vi "RH_Auto_with_Lockin_clear.vi"() -> ()   [LabVIEW 2019]
uses:
  <vilib>/Instr/_visa.llb/VISA Configure Serial Port (Instr).vi
  <vilib>/ptbypt/NI_PtbyPt.lvlib
panel:
  in  "0:OFF\n1:2.5mW\n2:25mW\n3:250mW\n4:2.5W\n5:25W":dbl=3.0
  in  "1:VTI 2:Sample":dbl=2.0
  in  "Termination Character":u8=10 format="%.0x"
  in  "Set VTI Heater Range":bool
  in  "Apply voltage":bool
  out "read buffer":string
  in  "Target [V]":string
  in  "start [V]":string
  in  "Keithley2400":refnum<visa-resource-name>="GPIB1::15::INSTR"
  out "Resistance [Ohm]":dbl=97.3586 format="%#_6f"
  out "Lockin y (V)":dbl=136.05
  out "Lockin x (V)":dbl=0.000139774
  in  "On:Delta\nOff:Lock-in":bool=TRUE
  in  "I for Lockin [A]":dbl=5e-06 format="%#_6e"
  out "Lockin Y (V)":dbl=-136.536
  out "Lockin X (V)":dbl=0.000486793
  in  "Lockin SR830":refnum<visa-resource-name>="GPIB1::8::INSTR"
  in  "T-ramp off":bool
  in  "Main sorb T control":bool
  in  "Wait [min]":i32
  in  "LakeShore335 (for He3)":refnum<visa-resource-name>="COM4"
  in  "Temp control off":bool
  out "temp [K]":dbl=1.4
  out "Waiting T-stability":bool caption="stabilizing"
  in  "Set Initial Field":bool
  in  "Field [T]":dbl
  in  "Period [s]":dbl=0.5 caption="Delay Time (s)"
  in  "Measure R-T":bool
  in  "Save R-T":bool
  out "R-T":cluster{"X":dbl[], "Y":dbl[]}[](graph) caption="XY Graph"
  out "Rate [K/min]":dbl=-0.11815951044220217 format="%#_6f"
  in  "Reset":bool
  in  "Stop":bool
  in  "Pause off":bool
  in  "Compliance [V]":dbl=0.5 format="%#_6f"
  out "R-H":cluster{"X":dbl[], "Y":dbl[]}[](graph) caption="XY Graph"
  in  "Reset":bool
  in  "Folder":path=path "C:/User Data/Graham" caption="Filename"
  out "Filename Out":path=path "C:/User Data/Bart/CG014_1012_3.00K"
  in  "File name":string="CG017a_3uA"
  out "VTI [K]":dbl=3.087
  out "VTI [K]":dbl=1.6151
  out "Sample Temp [K]":dbl=1.4
  out "Magnetic Field [T]":dbl=2.97271
  out "Delta reading [Ohm]":dbl
  out "Delta Reading [Ohm]":dbl=0.00314207515
  out "Sample Temp [K]":dbl=2.2127
  in  "Abort Delta":bool
  in  "Arm Delta":bool
  in  "DELAY [sec]":dbl=0.002 format="%#_6e"
  in  "I-HIGH [A]":dbl=0.0001 format="%#_6e"
  in  "Measure R-H":bool
  in  "Rate [K/min]":dbl=10.0
  in  "Set Temp [K]":dbl=1.0
  in  "Set Temperature":bool
  out "Magnetic Field [T]":dbl
  in  "Rate [T/min]":dbl=0.5
  in  "Set Field [T]":dbl
  in  "Set Field":bool
  in  "Keithley":refnum<visa-resource-name>="GPIB1::20::INSTR"
  in  "Skip":bool
  in  "Wait T-stable [min]":i32=30
  in  "period (s)":dbl=0.5 min=0.0 max=1111.0 step=0.1
  in  "stop 2":bool caption="Pause"
  in  "Wait field stable [sec]":dbl=20.0
  in  "Magnet Power supply":refnum<visa-resource-name>="COM6"
  in  "Set Field [T]   Rate [T/min]":dbl[][](array[numeric])=[[0.0, 0.2], [-6.0, 0.2], [0.0, 0.2], [6.0, 0.2]]
  in  "Set Temp [K]  Rate [K/min]":dbl[][](array[numeric])=[[10.0, 5.0], [0.0, 5.0], [0.0, 5.0], [0.0, 5.0], [0.0, 5.0]]
  in  "LakeShore340":refnum<visa-resource-name>="COM7"
  out "error out 3":errorcluster={"status"=FALSE, "code"=1073676294, "source"="VISA Read in RH_Auto_with_Lockin_clear.vi"}
  out "error out 2":errorcluster={"status"=FALSE, "code"=1073676294, "source"="VISA Read in RH_Auto_with_Lockin_clear.vi"}
  out "error out":errorcluster={"status"=FALSE, "code"=1073676294, "source"="VISA Read in RH_Auto_with_Lockin_clear.vi"}
  # "Manual control"
  # "R-H Auto Measurement"
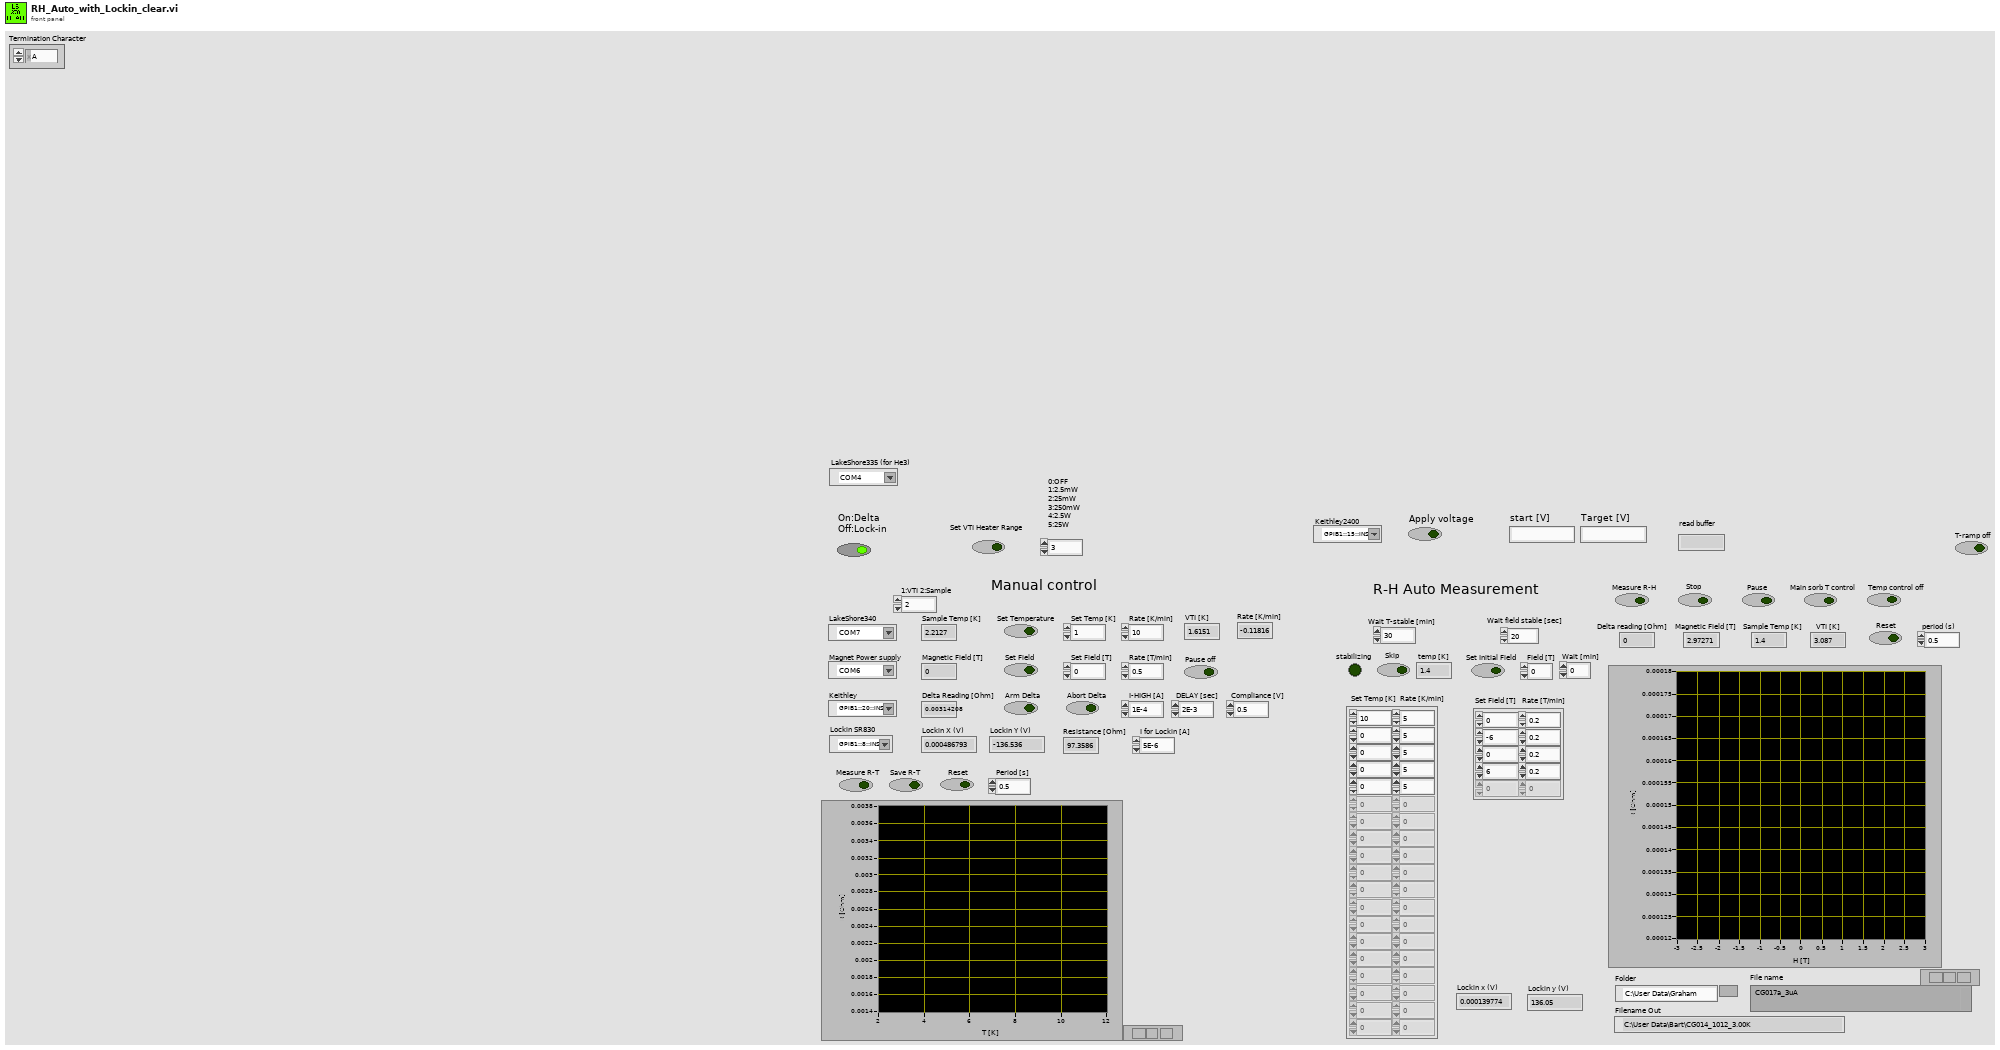
[diagram p1: front panel]
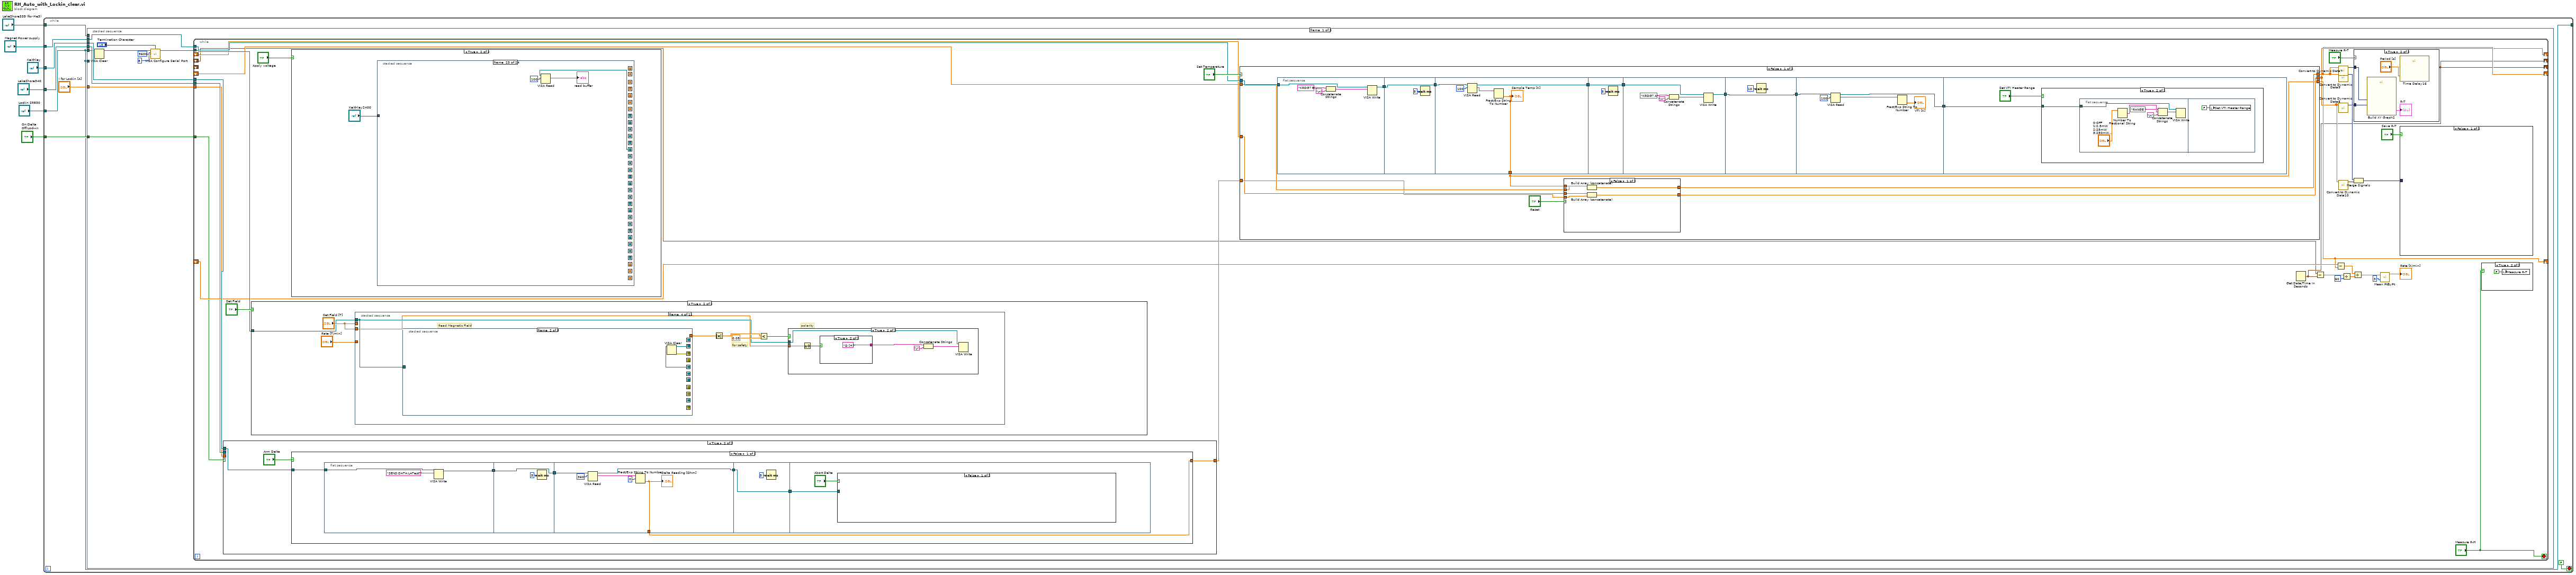
[diagram p0: block diagram]
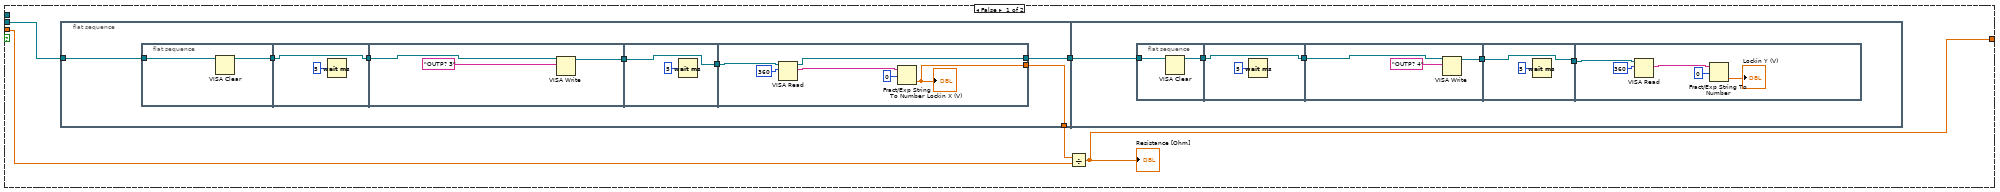
[diagram p2: hidden frame]
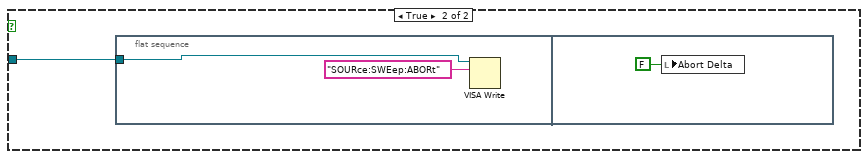
[diagram p3: hidden frame]
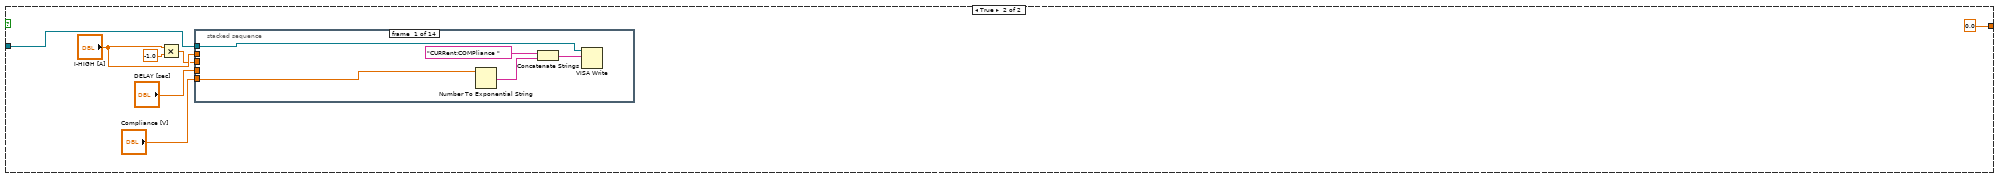
[diagram p4: hidden frame]
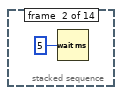
[diagram p5: hidden frame]
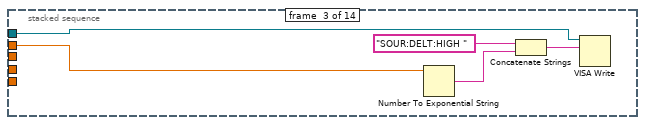
[diagram p6: hidden frame]
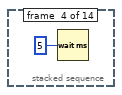
[diagram p7: hidden frame]
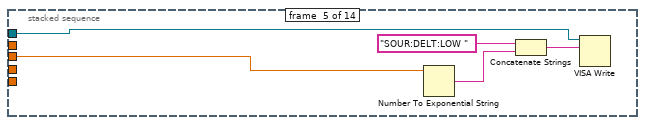
[diagram p8: hidden frame]
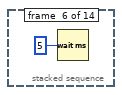
[diagram p9: hidden frame]
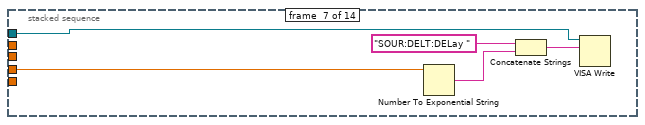
[diagram p10: hidden frame]
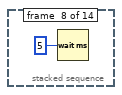
[diagram p11: hidden frame]
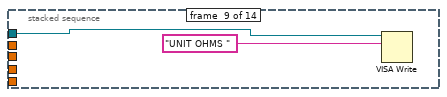
[diagram p12: hidden frame]
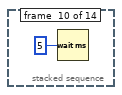
[diagram p13: hidden frame]
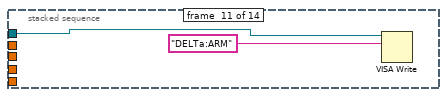
[diagram p14: hidden frame]
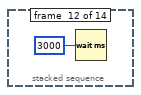
[diagram p15: hidden frame]
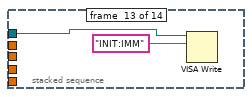
[diagram p16: hidden frame]
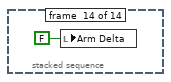
[diagram p17: hidden frame]
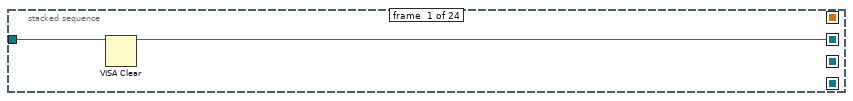
[diagram p19: hidden frame]
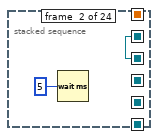
[diagram p20: hidden frame]
diagram:
  n1 = while {
    tunnel: "LakeShore340" -> [w14]
    tunnel: "Magnet Power supply" -> [w13]
    tunnel: "Keithley" -> [w12]
    tunnel: "LakeShore335 (for He3)" -> [w10]
    tunnel: "Lockin SR830" -> [w8]
    tunnel: "On:Delta\nOff:Lock-in" -> [w9]
    tunnel: [w8] -> _
    stop <- FALSE stop-if-true
    n2 = stacked-sequence {
      tunnel: w14 -> [w15 w534 _]
      tunnel: w13 -> [w25 w533 w1135]
      tunnel: w12 -> [w24 w532 _]
      tunnel: w10 -> [_ w530 _]
      tunnel: w8 -> [w23 _ _]
      tunnel: w9 -> [w22 w529 _]
      tunnel: w8 -> [_ w528 _]
      tunnel: "I for Lockin [A]" -> [w21 w527 _]
      frame #0 {
        n3 = VISA Clear(VISA resource name=w15) -> (VISA resource name out=w17:refnum<visa-resource-name>)  [unwired: 1 in, 1 out]
        n4 = call-poly "VISA Configure Serial Port"("VISA resource name"=w17, "termination char\n(0xA = '\\n' = LF)"="Termination Character", "baud rate (9600)"=9600, "data bits (8)"=8) -> ("VISA resource name out"=w16:refnum<visa-resource-name>)  [unwired: 10 in, 1 out]
        n5 = while {
          tunnel: w25 -> [w54]
          tunnel: w16 -> [w56]
          tunnel: w24 -> [w55]
          shift-right: [w42] -> _
          shift-left: _ -> [w37]
          shift-right: [w40] -> _
          shift-left: _ -> [w52]
          shift-right: [w34] -> _
          shift-left: _ -> [_]
          shift-right: [w50] -> _
          shift-left: _ -> [w51]
          shift-right: [w34] -> _
          shift-left: _ -> [w33]
          tunnel: w23 -> [w29]
          tunnel: w22 -> [w28]
          tunnel: w21 -> [w26]
          stop <- "Measure R-H" stop-if-true
          n6 = case shown="True" w28 {
            tunnel: w55 -> [_ w107]
            tunnel: [w61 w105] -> w53
            tunnel: w29 -> [w62 _]
            tunnel: w26 -> [w59 _]
            frame False {
              n7 = flat-sequence {
                tunnel: [w68] -> w63
                tunnel: w62 -> [w67]
                tunnel: [w64] -> w60
                tunnel: w60 -> [w86]
                frame #0 {
                  n8 = flat-sequence {
                    tunnel: w67 -> [w72]
                    tunnel: [w71] -> w65
                    tunnel: [w74] -> w66
                    tunnel: w65 -> [w74]
                    tunnel: [w75] -> w70
                    tunnel: w66 -> [w77]
                    tunnel: [w78] -> w69
                    tunnel: w70 -> [w78]
                    tunnel: w69 -> [w83]
                    tunnel: [w81] -> w68
                    tunnel: [w80] -> w64
                    frame #0 {
                      n9 = VISA Clear(VISA resource name=w72) -> (VISA resource name out=w71:refnum<visa-resource-name>)  [unwired: 1 in, 1 out]
                    }
                    frame #1 {
                      n10 = Wait (ms)(milliseconds to wait=5) -> ()  [unwired: 1 out]
                    }
                    frame #2 {
                      n11 = VISA Write(VISA resource name=w77, write buffer="OUTP? 3" ("write buffer 2")) -> (VISA resource name out=w75:refnum<visa-resource-name>)  [unwired: 1 in, 2 out]
                    }
                    frame #3 {
                      n12 = Wait (ms)(milliseconds to wait=5) -> ()  [unwired: 1 out]
                    }
                    frame #4 {
                      n13 = VISA Read(VISA resource name=w83, byte count=u32 360) -> (VISA resource name out=w80:refnum<visa-resource-name>, read buffer=w82:string)  [unwired: 1 in, 2 out]
                      n14 = Fract/Exp String To Number(string=w82, offset=0) -> (number=w81:dbl)  [unwired: 3 out]
                      "Lockin X (V)" <- w81
                    }
                  }
                }
                frame #1 {
                  n15 = flat-sequence {
                    tunnel: w86 -> [w92]
                    tunnel: [w91] -> w87
                    tunnel: [w94] -> w88
                    tunnel: w87 -> [w94]
                    tunnel: [w95] -> w90
                    tunnel: w88 -> [w97]
                    tunnel: [w98] -> w89
                    tunnel: w90 -> [w98]
                    tunnel: w89 -> [w102]
                    frame #0 {
                      n16 = VISA Clear(VISA resource name=w92) -> (VISA resource name out=w91:refnum<visa-resource-name>)  [unwired: 1 in, 1 out]
                    }
                    frame #1 {
                      n17 = Wait (ms)(milliseconds to wait=5) -> ()  [unwired: 1 out]
                    }
                    frame #2 {
                      n18 = VISA Write(VISA resource name=w97, write buffer="OUTP? 4" ("write buffer 2")) -> (VISA resource name out=w95:refnum<visa-resource-name>)  [unwired: 1 in, 2 out]
                    }
                    frame #3 {
                      n19 = Wait (ms)(milliseconds to wait=5) -> ()  [unwired: 1 out]
                    }
                    frame #4 {
                      n20 = VISA Read(VISA resource name=w102, byte count=u32 360) -> (read buffer=w101:string)  [unwired: 1 in, 3 out]
                      n21 = Fract/Exp String To Number(string=w101, offset=0) -> (number=→"Lockin Y (V)":dbl)  [unwired: 3 out]
                    }
                  }
                }
              }
              n22 = Divide(x=w63, y=w59) -> (x/y=w61:dbl)
              "Resistance [Ohm]" <- w61
            }
            frame True {
              n23 = case shown="False" "Arm Delta" {
                tunnel: w107 -> [w113 w137]
                tunnel: [w108 0.0] -> w105
                frame False {
                  n24 = flat-sequence {
                    tunnel: w113 -> [w116]
                    tunnel: [w114] -> w111
                    tunnel: [w117] -> w112
                    tunnel: w111 -> [w117]
                    tunnel: w112 -> [w121]
                    tunnel: [w120] -> w109
                    tunnel: [w119] -> w108
                    tunnel: [w125] -> w110
                    tunnel: w109 -> [w125]
                    tunnel: w110 -> [w127]
                    frame #0 {
                      n25 = VISA Write(VISA resource name=w116, write buffer="SENS:DATA:LATest?" ("write buffer 2")) -> (VISA resource name out=w114:refnum<visa-resource-name>)  [unwired: 1 in, 2 out]
                    }
                    frame #1 {
                      n26 = Wait (ms)(milliseconds to wait=5) -> ()  [unwired: 1 out]
                    }
                    frame #2 {
                      n27 = VISA Read(VISA resource name=w121, byte count=u32 360) -> (VISA resource name out=w120:refnum<visa-resource-name>, read buffer=w123:string)  [unwired: 1 in, 2 out]
                      n28 = Fract/Exp String To Number(string=w123, offset=0) -> (number=w119:dbl)  [unwired: 3 out]
                      "Delta Reading [Ohm]" <- w119
                    }
                    frame #3 {
                      n29 = Wait (ms)(milliseconds to wait=5) -> ()  [unwired: 1 out]
                    }
                    frame #4 {
                      n30 = case shown="False" "Abort Delta" {
                        tunnel: w127 -> [_ w129]
                        frame False {
                        }
                        frame True {
                          n31 = flat-sequence {
                            tunnel: w129 -> [w131]
                            frame #0 {
                              n32 = VISA Write(VISA resource name=w131, write buffer="SOURce:SWEep:ABORt") -> ()  [unwired: 1 in, 3 out]
                            }
                            frame #1 {
                              n33 = local write "Abort Delta"(FALSE) -> ()
                            }
                          }
                        }
                      }
                    }
                  }
                }
                frame True {
                  n34 = Multiply(x="I-HIGH [A]", y=-1.0) -> (x*y=w136:dbl)
                  n35 = stacked-sequence {
                    tunnel: "I-HIGH [A]" -> [_ _ w148 _ _ _ _ _ _ _ _ _ _ _]
                    tunnel: w137 -> [w141 _ w146 _ w153 _ w159 _ w164 _ w167 _ w170 _]
                    tunnel: w136 -> [_ _ _ _ w152 _ _ _ _ _ _ _ _ _]
                    tunnel: "DELAY [sec]" -> [_ _ _ _ _ _ w158 _ _ _ _ _ _ _]
                    tunnel: "Compliance [V]" -> [w140 _ _ _ _ _ _ _ _ _ _ _ _ _]
                    frame #0 {
                      n36 = Number To Exponential String(number=w140) -> (E-format string=w143:string)  [unwired: 3 in]
                      n37 = Concatenate Strings("CURRent:COMPliance ", w143) -> (w142:string)
                      n38 = VISA Write(VISA resource name=w141, write buffer=w142) -> ()  [unwired: 1 in, 3 out]
                    }
                    frame #1 {
                      n39 = Wait (ms)(milliseconds to wait=5) -> ()  [unwired: 1 out]
                    }
                    frame #2 {
                      n40 = Number To Exponential String(number=w148) -> (E-format string=w149:string)  [unwired: 3 in]
                      n41 = Concatenate Strings("SOUR:DELT:HIGH ", w149) -> (w147:string)
                      n42 = VISA Write(VISA resource name=w146, write buffer=w147) -> ()  [unwired: 1 in, 3 out]
                    }
                    frame #3 {
                      n43 = Wait (ms)(milliseconds to wait=5) -> ()  [unwired: 1 out]
                    }
                    frame #4 {
                      n44 = Number To Exponential String(number=w152) -> (E-format string=w155:string)  [unwired: 3 in]
                      n45 = Concatenate Strings("SOUR:DELT:LOW ", w155) -> (w154:string)
                      n46 = VISA Write(VISA resource name=w153, write buffer=w154) -> ()  [unwired: 1 in, 3 out]
                    }
                    frame #5 {
                      n47 = Wait (ms)(milliseconds to wait=5) -> ()  [unwired: 1 out]
                    }
                    frame #6 {
                      n48 = Number To Exponential String(number=w158) -> (E-format string=w161:string)  [unwired: 3 in]
                      n49 = Concatenate Strings("SOUR:DELT:DELay ", w161) -> (w160:string)
                      n50 = VISA Write(VISA resource name=w159, write buffer=w160) -> ()  [unwired: 1 in, 3 out]
                    }
                    frame #7 {
                      n51 = Wait (ms)(milliseconds to wait=5) -> ()  [unwired: 1 out]
                    }
                    frame #8 {
                      n52 = VISA Write(VISA resource name=w164, write buffer="UNIT OHMS ") -> ()  [unwired: 1 in, 3 out]
                    }
                    frame #9 {
                      n53 = Wait (ms)(milliseconds to wait=5) -> ()  [unwired: 1 out]
                    }
                    frame #10 {
                      n54 = VISA Write(VISA resource name=w167, write buffer="DELTa:ARM") -> ()  [unwired: 1 in, 3 out]
                    }
                    frame #11 {
                      n55 = Wait (ms)(milliseconds to wait=3000) -> ()  [unwired: 1 out]
                    }
                    frame #12 {
                      n56 = VISA Write(VISA resource name=w170, write buffer="INIT:IMM") -> ()  [unwired: 1 in, 3 out]
                    }
                    frame #13 {
                      n57 = local write "Arm Delta"(FALSE) -> ()
                    }
                  }
                }
              }
            }
          }
          n58 = case shown="True" "Set Field" {
            tunnel: w54 -> [w362 w432]
            frame False {
              n59 = stacked-sequence {
                seq-local: [w363 _ _ _ _ _ _ _] -> [_ w366 _ _ _ _ _ _]
                seq-local: [_ w364 _ _ _ _ _ _] -> [_ _ w370 _ _ _ _ _]
                seq-local: [_ w365 _ _ _ _ _ _] -> [_ _ w367 _ _ _ _ _]
                seq-local: [_ _ w369 _ _ _ _ _] -> [_ _ _ w410 _ _ _ _]
                seq-local: [_ _ w368 _ _ _ _ _] -> [_ _ _ w409 _ _ _ _]
                seq-local: [_ _ _ w412 _ _ _ _] -> [_ _ _ _ w415 _ _ _]
                seq-local: [_ _ _ w411 _ _ _ _] -> [_ _ _ _ w416 _ _ _]
                seq-local: [_ _ _ _ w415 _ _ _] -> [_ _ _ _ _ w427 _ _]
                seq-local: [_ _ _ _ w416 _ _ _] -> [_ _ _ _ _ w425 _ _]
                seq-local: [_ _ _ _ _ w426 _ _] -> [_ _ _ _ _ _ _ w431]
                seq-local: [_ _ _ _ _ w424 _ _] -> [_ _ _ _ _ _ _ w430]
                tunnel: w362 -> [w363 _ _ _ _ _ _ _]
                tunnel: [_ _ _ _ _ w417 _ _] -> w361
                frame #0 {
                }
                frame #1 {
                  n60 = VISA Clear(VISA resource name=w366) -> (VISA resource name out=w364:refnum<visa-resource-name>, error out=w365:errorcluster)  [unwired: 1 in]
                }
                frame #2 {
                  n61 = flat-sequence {
                    tunnel: w370 -> [w374]
                    tunnel: [w373] -> w369
                    tunnel: [w372] -> w368
                    tunnel: w367 -> [w371]
                    frame #0 {
                      n62 = call "Time Delay8"() -> ()  [unwired: 11 in, 1 out]
                    }
                    frame #1 {
                      n63 = case shown="False" "Pause off" {
                        tunnel: w374 -> [w377 w389]
                        tunnel: [w377 w378] -> w373
                        tunnel: [w376 w381] -> w372
                        tunnel: w371 -> [w376 w384]
                        frame False {
                        }
                        frame True {
                          n64 = flat-sequence {
                            tunnel: w389 -> [w393]
                            tunnel: [w392] -> w387
                            tunnel: [w391] -> w385
                            tunnel: w384 -> [w390]
                            tunnel: [w398] -> w388
                            tunnel: w387 -> [w398]
                            tunnel: [w397] -> w386
                            tunnel: w385 -> [w397]
                            tunnel: w388 -> [w400]
                            tunnel: w386 -> [_]
                            tunnel: [w400] -> w383
                            tunnel: [w399] -> w379
                            tunnel: w383 -> [w402]
                            tunnel: [w402] -> w382
                            tunnel: [w401] -> w380
                            tunnel: w379 -> [w401]
                            tunnel: [w406] -> w378
                            tunnel: w382 -> [w405]
                            tunnel: [w404] -> w381
                            tunnel: w380 -> [w403]
                            frame #0 {
                              n65 = Concatenate Strings("P 0" ("Command"), "\r") -> (w395:string)
                              n66 = VISA Write(VISA resource name=w393, write buffer=w395, error in (no error)=w390) -> (VISA resource name out=w392:refnum<visa-resource-name>, error out=w391:errorcluster)  [unwired: 1 out]
                            }
                            frame #1 {
                              n67 = call "Time Delay14"() -> ()  [unwired: 11 in, 1 out]
                            }
                            frame #2 {
                              n68 = VISA Close(VISA resource name=w400) -> (error out=w399:errorcluster)  [unwired: 1 in]
                            }
                            frame #3 {
                              n69 = call "Time Delay15"() -> ()  [unwired: 11 in, 1 out]
                            }
                            frame #4 {
                              n70 = VISA Clear(VISA resource name=w405, error in (no error)=w403) -> (VISA resource name out=w406:refnum<visa-resource-name>, error out=w404:errorcluster)
                            }
                            frame #5 {
                              n71 = local write "Pause off"(FALSE) -> ()
                            }
                          }
                        }
                      }
                    }
                  }
                }
                frame #3 {
                  n72 = Concatenate Strings("G O" ("Command"), "\r") -> (w413:string)
                  n73 = VISA Write(VISA resource name=w410, write buffer=w413, error in (no error)=w409) -> (VISA resource name out=w412:refnum<visa-resource-name>, error out=w411:errorcluster)  [unwired: 1 out]
                }
                frame #4 {
                  n74 = call "Time Delay9"() -> ()  [unwired: 11 in, 1 out]
                }
                frame #5 {
                  n75 = VISA Read(VISA resource name=w427, byte count=u32 30, error in (no error)=w425) -> (VISA resource name out=w426:refnum<visa-resource-name>, read buffer=w421:string, error out=w424:errorcluster)  [unwired: 1 out]
                  n76 = Match Pattern(string=w421, regular expression="OUTPUT:") -> (after substring=w419:string)  [unwired: 1 in, 3 out]
                  n77 = Match Pattern(string=w419, regular expression=" TESLA") -> (before substring=w418:string)  [unwired: 1 in, 3 out]
                  n78 = Fract/Exp String To Number(string=w418, offset=0) -> (number=w417:dbl)  [unwired: 2 in, 1 out]
                }
                frame #6 {
                  n79 = call "Time Delay10"() -> ()  [unwired: 11 in, 1 out]
                }
                frame #7 {
                  n80 = VISA Close(VISA resource name=w431, error in (no error)=w430) -> (error out=→"error out":errorcluster)
                }
              }
              "Magnetic Field [T]" <- w361
            }
            frame True {
              n81 = stacked-sequence {
                tunnel: w432 -> [w435 _ _ w454 _ w499 _ w517 _ w522 _]
                tunnel: "Set Field [T]" -> [_ w437 _ _ _ _ _ _ _ _ _]
                tunnel: "Rate [T/min]" -> [_ w436 _ _ _ _ _ w507 _ _ _]
                tunnel: "Set Field [T]" -> [_ _ _ w453 _ w497 _ _ _ _ _]
                frame #0 {
                  n82 = VISA Clear(VISA resource name=w435) -> ()  [unwired: 1 in, 2 out]
                }
                frame #1 {
                  n83 = Greater?(x=w437, y=10) -> (0:w438:bool)
                  n84 = Greater?(x=w436, y=0.6) -> (0:w447:bool)
                  n85 = Less?(x=w437, y=-10) -> (x < y?=w443:bool)
                  n86 = Less?(x=w436, y=-0.6) -> (x < y?=w446:bool)
                  n87 = Or(x=w438, y=w443) -> (x .or. y?=w449:bool)
                  n88 = Or(x=w447, y=w446) -> (x .or. y?=w448:bool)
                  n89 = call "Display Message to User6"("Enable"=w449) -> ("OK"=w450:bool)  [unwired: 9 in, 1 out]
                  n90 = call "Display Message to User5"("Enable"=w448) -> ("OK"=w439:bool)  [unwired: 9 in, 1 out]
                  n91 = Or(x=w450, y=w439) -> (x .or. y?=w440:bool)
                  n92 = Stop(stop? (T)=w440) -> ()
                }
                frame #2 {
                  n93 = Wait (ms)(milliseconds to wait=500) -> ()  [unwired: 1 out]
                }
                frame #3 {
                  # "Read Magnetic Field"
                  # "for safety"
                  # "polarity"
                  n94 = stacked-sequence {
                    seq-local: [w458 _ _ _ _ _ _ _] -> [_ w461 _ _ _ _ _ _]
                    seq-local: [_ w459 _ _ _ _ _ _] -> [_ _ w463 _ _ _ _ _]
                    seq-local: [_ w460 _ _ _ _ _ _] -> [_ _ w462 _ _ _ _ _]
                    seq-local: [_ _ w463 _ _ _ _ _] -> [_ _ _ w466 _ _ _ _]
                    seq-local: [_ _ w462 _ _ _ _ _] -> [_ _ _ w465 _ _ _ _]
                    seq-local: [_ _ _ w468 _ _ _ _] -> [_ _ _ _ w471 _ _ _]
                    seq-local: [_ _ _ w467 _ _ _ _] -> [_ _ _ _ w472 _ _ _]
                    seq-local: [_ _ _ _ w471 _ _ _] -> [_ _ _ _ _ w483 _ _]
                    seq-local: [_ _ _ _ w472 _ _ _] -> [_ _ _ _ _ w481 _ _]
                    seq-local: [_ _ _ _ _ w482 _ _] -> [_ _ _ _ _ _ _ w487]
                    seq-local: [_ _ _ _ _ w480 _ _] -> [_ _ _ _ _ _ _ w486]
                    tunnel: w454 -> [w458 _ _ _ _ _ _ _]
                    tunnel: [_ _ _ _ _ w473 _ _] -> w455
                    frame #0 {
                    }
                    frame #1 {
                      n95 = VISA Clear(VISA resource name=w461) -> (VISA resource name out=w459:refnum<visa-resource-name>, error out=w460:errorcluster)  [unwired: 1 in]
                    }
                    frame #2 {
                      n96 = call "Time Delay6"() -> ()  [unwired: 11 in, 1 out]
                    }
                    frame #3 {
                      n97 = Concatenate Strings("G O" ("Command"), "\r") -> (w469:string)
                      n98 = VISA Write(VISA resource name=w466, write buffer=w469, error in (no error)=w465) -> (VISA resource name out=w468:refnum<visa-resource-name>, error out=w467:errorcluster)  [unwired: 1 out]
                    }
                    frame #4 {
                      n99 = call "Time Delay7"() -> ()  [unwired: 11 in, 1 out]
                    }
                    frame #5 {
                      n100 = VISA Read(VISA resource name=w483, byte count=u32 30, error in (no error)=w481) -> (VISA resource name out=w482:refnum<visa-resource-name>, read buffer=w477:string, error out=w480:errorcluster)  [unwired: 1 out]
                      n101 = Match Pattern(string=w477, regular expression="OUTPUT:") -> (after substring=w475:string)  [unwired: 1 in, 3 out]
                      n102 = Match Pattern(string=w475, regular expression=" TESLA") -> (before substring=w474:string)  [unwired: 1 in, 3 out]
                      n103 = Fract/Exp String To Number(string=w474, offset=0) -> (number=w473:dbl)  [unwired: 2 in, 1 out]
                    }
                    frame #6 {
                      n104 = call "Time Delay11"() -> ()  [unwired: 11 in, 1 out]
                    }
                    frame #7 {
                      n105 = VISA Close(VISA resource name=w487, error in (no error)=w486) -> (error out=→"error out 2":errorcluster)
                    }
                  }
                  n106 = Absolute Value(x=w455) -> (abs(x)=w456:dbl)
                  n107 = Less?(x=w456, y=0.05) -> (x < y?=w452:bool)
                  n108 = case shown="True" w452 {
                    tunnel: w454 -> [_ w490]
                    tunnel: w453 -> [_ w488]
                    frame False {
                    }
                    frame True {
                      n109 = Greater Or Equal To 0?(x=w488) -> (x >= 0?=w489:bool)
                      n110 = case shown="True" w489 {
                        tunnel: ["D [-]" ("data") "D [+]" ("data")] -> w491
                        frame False {
                        }
                        frame True {
                        }
                      }
                      n111 = Concatenate Strings(w491, "\r") -> (w493:string)
                      n112 = VISA Write(VISA resource name=w490, write buffer=w493) -> ()  [unwired: 1 in, 3 out]
                    }
                  }
                }
                frame #4 {
                  n113 = Wait (ms)(milliseconds to wait=500) -> ()  [unwired: 1 out]
                }
                frame #5 {
                  # "set set field"
                  n114 = Number To Fractional String(number=w497, width (-)=i16 6, precision (6)=i16 3) -> (F-format string=w502:string)  [unwired: 1 in]
                  n115 = Concatenate Strings("S [%][MID] " ("string"), w502) -> (w498:string)
                  n116 = Concatenate Strings(w498, "\r") -> (w501:string)
                  n117 = VISA Write(VISA resource name=w499, write buffer=w501) -> ()  [unwired: 1 in, 3 out]
                }
                frame #6 {
                  n118 = Wait (ms)(milliseconds to wait=500) -> ()  [unwired: 1 out]
                }
                frame #7 {
                  # "set rate"
                  n119 = Divide(x=w507, y=60.0) -> (x/y=w512:dbl)
                  n120 = Divide(x=w512, y=0.09797) -> (x/y=w510:dbl)
                  n121 = Number To Fractional String(number=w510, width (-)=i16 6, precision (6)=i16 3) -> (F-format string=w515:string)  [unwired: 1 in]
                  n122 = Concatenate Strings("S R " ("string"), w515) -> (w514:string)
                  n123 = Concatenate Strings(w514, "\r") -> (w519:string)
                  n124 = VISA Write(VISA resource name=w517, write buffer=w519) -> ()  [unwired: 1 in, 3 out]
                }
                frame #8 {
                  n125 = Wait (ms)(milliseconds to wait=500) -> ()  [unwired: 1 out]
                }
                frame #9 {
                  # "Go to set field"
                  n126 = Concatenate Strings("R [%][MID]" ("data"), "\r") -> (w524:string)
                  n127 = VISA Write(VISA resource name=w522, write buffer=w524) -> ()  [unwired: 1 in, 3 out]
                }
                frame #10 {
                  n128 = local write "Set Field"(FALSE) -> ()
                  n129 = Wait (ms)(milliseconds to wait=500) -> ()  [unwired: 1 out]
                }
              }
            }
          }
          n130 = case shown="True" "Apply voltage" {
            frame False {
            }
            frame True {
              n131 = stacked-sequence {
                seq-local: [w174 _ _ _ _ _ _ _ _ _ _ _ _ _ _ _ _ _ _ _ _ _ _ _] -> [_ w177 _ _ _ _ _ _ _ _ _ _ _ _ _ _ _ _ _ _ _ _ _ _]
                seq-local: [_ w177 _ _ _ _ _ _ _ _ _ _ _ _ _ _ _ _ _ _ _ _ _ _] -> [_ _ w180 _ _ _ _ _ _ _ _ _ _ _ _ _ _ _ _ _ _ _ _ _]
                seq-local: [_ _ w179 _ _ _ _ _ _ _ _ _ _ _ _ _ _ _ _ _ _ _ _ _] -> [_ _ _ w182 _ _ _ _ _ _ _ _ _ _ _ _ _ _ _ _ _ _ _ _]
                seq-local: [_ _ _ w182 _ _ _ _ _ _ _ _ _ _ _ _ _ _ _ _ _ _ _ _] -> [_ _ _ _ w184 _ _ _ _ _ _ _ _ _ _ _ _ _ _ _ _ _ _ _]
                seq-local: [_ _ _ _ w183 _ _ _ _ _ _ _ _ _ _ _ _ _ _ _ _ _ _ _] -> [_ _ _ _ _ w187 _ _ _ _ _ _ _ _ _ _ _ _ _ _ _ _ _ _]
                seq-local: [_ _ _ _ _ w187 _ _ _ _ _ _ _ _ _ _ _ _ _ _ _ _ _ _] -> [_ _ _ _ _ _ w189 _ _ _ _ _ _ _ _ _ _ _ _ _ _ _ _ _]
                seq-local: [_ _ _ _ _ _ w188 _ _ _ _ _ _ _ _ _ _ _ _ _ _ _ _ _] -> [_ _ _ _ _ _ _ w191 _ _ _ _ _ _ _ _ _ _ _ _ _ _ _ _]
                seq-local: [_ _ _ _ _ _ _ w191 _ _ _ _ _ _ _ _ _ _ _ _ _ _ _ _] -> [_ _ _ _ _ _ _ _ w194 _ _ _ _ _ _ _ _ _ _ _ _ _ _ _]
                seq-local: [_ _ _ _ _ _ _ _ w193 _ _ _ _ _ _ _ _ _ _ _ _ _ _ _] -> [_ _ _ _ _ _ _ _ _ w196 _ _ _ _ _ _ _ _ _ _ _ _ _ _]
                seq-local: [_ _ _ _ _ _ _ _ _ w196 _ _ _ _ _ _ _ _ _ _ _ _ _ _] -> [_ _ _ _ _ _ _ _ _ _ w203 _ _ _ _ _ _ _ _ _ _ _ _ _]
                seq-local: [_ _ _ _ _ _ _ _ _ _ w202 _ _ _ _ _ _ _ _ _ _ _ _ _] -> [_ _ _ _ _ _ _ _ _ _ _ w205 _ _ _ _ _ _ _ _ _ _ _ _]
                seq-local: [_ _ _ _ _ _ _ _ _ _ w198 _ _ _ _ _ _ _ _ _ _ _ _ _] -> [_ _ _ _ _ _ _ _ _ _ _ w204 _ _ _ _ _ _ _ _ _ _ _ _]
                seq-local: [_ _ _ _ _ _ _ _ _ _ _ w205 _ _ _ _ _ _ _ _ _ _ _ _] -> [_ _ _ _ _ _ _ _ _ _ _ _ w213 _ _ _ _ _ _ _ _ _ _ _]
                seq-local: [_ _ _ _ _ _ _ _ _ _ _ w204 _ _ _ _ _ _ _ _ _ _ _ _] -> [_ _ _ _ _ _ _ _ _ _ _ _ w207 _ _ _ _ _ _ _ _ _ _ _]
                seq-local: [_ _ _ _ _ _ _ _ _ _ _ _ w212 _ _ _ _ _ _ _ _ _ _ _] -> [_ _ _ _ _ _ _ _ _ _ _ _ _ w216 _ _ _ _ _ _ _ _ _ _]
                seq-local: [_ _ _ _ _ _ _ _ _ _ _ _ w208 _ _ _ _ _ _ _ _ _ _ _] -> [_ _ _ _ _ _ _ _ _ _ _ _ _ w215 _ _ _ _ _ _ _ _ _ _]
                seq-local: [_ _ _ _ _ _ _ _ _ _ _ _ w207 _ _ _ _ _ _ _ _ _ _ _] -> [_ _ _ _ _ _ _ _ _ _ _ _ _ w214 _ _ _ _ _ _ _ _ _ _]
                seq-local: [_ _ _ _ _ _ _ _ _ _ _ _ _ w216 _ _ _ _ _ _ _ _ _ _] -> [_ _ _ _ _ _ _ _ _ _ _ _ _ _ w225 _ _ _ _ _ _ _ _ _]
                seq-local: [_ _ _ _ _ _ _ _ _ _ _ _ _ w215 _ _ _ _ _ _ _ _ _ _] -> [_ _ _ _ _ _ _ _ _ _ _ _ _ _ w219 _ _ _ _ _ _ _ _ _]
                seq-local: [_ _ _ _ _ _ _ _ _ _ _ _ _ w214 _ _ _ _ _ _ _ _ _ _] -> [_ _ _ _ _ _ _ _ _ _ _ _ _ _ w218 _ _ _ _ _ _ _ _ _]
                seq-local: [_ _ _ _ _ _ _ _ _ _ _ _ _ _ w224 _ _ _ _ _ _ _ _ _] -> [_ _ _ _ _ _ _ _ _ _ _ _ _ _ _ w231 _ _ _ _ _ _ _ _]
                seq-local: [_ _ _ _ _ _ _ _ _ _ _ _ _ _ w219 _ _ _ _ _ _ _ _ _] -> [_ _ _ _ _ _ _ _ _ _ _ _ _ _ _ w229 _ _ _ _ _ _ _ _]
                seq-local: [_ _ _ _ _ _ _ _ _ _ _ _ _ _ w218 _ _ _ _ _ _ _ _ _] -> [_ _ _ _ _ _ _ _ _ _ _ _ _ _ _ w228 _ _ _ _ _ _ _ _]
                seq-local: [_ _ _ _ _ _ _ _ _ _ _ _ _ _ _ w231 _ _ _ _ _ _ _ _] -> [_ _ _ _ _ _ _ _ _ _ _ _ _ _ _ _ w242 _ _ _ _ _ _ _]
                seq-local: [_ _ _ _ _ _ _ _ _ _ _ _ _ _ _ w229 _ _ _ _ _ _ _ _] -> [_ _ _ _ _ _ _ _ _ _ _ _ _ _ _ _ w240 _ _ _ _ _ _ _]
                seq-local: [_ _ _ _ _ _ _ _ _ _ _ _ _ _ _ w228 _ _ _ _ _ _ _ _] -> [_ _ _ _ _ _ _ _ _ _ _ _ _ _ _ _ w239 _ _ _ _ _ _ _]
                seq-local: [_ _ _ _ _ _ _ _ _ _ _ _ _ _ _ _ w241 _ _ _ _ _ _ _] -> [_ _ _ _ _ _ _ _ _ _ _ _ _ _ _ _ _ w244 _ _ _ _ _ _]
                seq-local: [_ _ _ _ _ _ _ _ _ _ _ _ _ _ _ _ _ w244 _ _ _ _ _ _] -> [_ _ _ _ _ _ _ _ _ _ _ _ _ _ _ _ _ _ w246 _ _ _ _ _]
                seq-local: [_ _ _ _ _ _ _ _ _ _ _ _ _ _ _ _ _ _ w245 _ _ _ _ _] -> [_ _ _ _ _ _ _ _ _ _ _ _ _ _ _ _ _ _ _ w249 _ _ _ _]
                seq-local: [_ _ _ _ _ _ _ _ _ _ _ _ _ _ _ _ _ _ _ w249 _ _ _ _] -> [_ _ _ _ _ _ _ _ _ _ _ _ _ _ _ _ _ _ _ _ w251 _ _ _]
                seq-local: [_ _ _ _ _ _ _ _ _ _ _ _ _ _ _ _ _ _ _ _ w250 _ _ _] -> [_ _ _ _ _ _ _ _ _ _ _ _ _ _ _ _ _ _ _ _ _ w253 _ _]
                seq-local: [_ _ _ _ _ _ _ _ _ _ _ _ _ _ _ _ _ _ _ _ _ w253 _ _] -> [_ _ _ _ _ _ _ _ _ _ _ _ _ _ _ _ _ _ _ _ _ _ w257 _]
                tunnel: "Keithley2400" -> [w175 _ _ _ _ _ _ _ _ _ _ _ _ _ _ _ _ _ _ _ _ _ _ _]
                frame #0 {
                  n132 = VISA Clear(VISA resource name=w175) -> (VISA resource name out=w174:refnum<visa-resource-name>)  [unwired: 1 in, 1 out]
                }
                frame #1 {
                  n133 = Wait (ms)(milliseconds to wait=u32 5) -> ()  [unwired: 1 out]
                }
                frame #2 {
                  n134 = VISA Write(VISA resource name=w180, write buffer=":SOUR:VOLT 0" ("write buffer 2")) -> (VISA resource name out=w179:refnum<visa-resource-name>)  [unwired: 1 in, 2 out]
                }
                frame #3 {
                  n135 = Wait (ms)(milliseconds to wait=u32 5) -> ()  [unwired: 1 out]
                }
                frame #4 {
                  n136 = VISA Write(VISA resource name=w184, write buffer=":SOUR:DEL 0.1" ("write buffer 2")) -> (VISA resource name out=w183:refnum<visa-resource-name>)  [unwired: 1 in, 2 out]
                }
                frame #5 {
                  n137 = Wait (ms)(milliseconds to wait=u32 5) -> ()  [unwired: 1 out]
                }
                frame #6 {
                  n138 = VISA Write(VISA resource name=w189, write buffer=":SOUR:VOLT:MODE SWE" ("write buffer 2")) -> (VISA resource name out=w188:refnum<visa-resource-name>)  [unwired: 1 in, 2 out]
                }
                frame #7 {
                  n139 = Wait (ms)(milliseconds to wait=u32 5) -> ()  [unwired: 1 out]
                }
                frame #8 {
                  n140 = VISA Write(VISA resource name=w194, write buffer=":SOUR:SWE:SPAC LIN" ("write buffer 2")) -> (VISA resource name out=w193:refnum<visa-resource-name>)  [unwired: 1 in, 2 out]
                }
                frame #9 {
                  n141 = Wait (ms)(milliseconds to wait=u32 5) -> ()  [unwired: 1 out]
                }
                frame #10 {
                  n142 = Fract/Exp String To Number(string="start [V]") -> (number=w198:dbl)  [unwired: 3 in, 1 out]
                  n143 = Concatenate Strings(":SOUR:VOLT:STAR " ("write buffer 2"), "start [V]") -> (w200:string)
                  n144 = VISA Write(VISA resource name=w203, write buffer=w200) -> (VISA resource name out=w202:refnum<visa-resource-name>)  [unwired: 1 in, 2 out]
                }
                frame #11 {
                  n145 = Wait (ms)(milliseconds to wait=u32 5) -> ()  [unwired: 1 out]
                }
                frame #12 {
                  n146 = Fract/Exp String To Number(string="Target [V]") -> (number=w208:dbl)  [unwired: 3 in, 1 out]
                  n147 = Concatenate Strings(":SOUR:VOLT:STOP " ("write buffer 2"), "Target [V]") -> (w210:string)
                  n148 = VISA Write(VISA resource name=w213, write buffer=w210) -> (VISA resource name out=w212:refnum<visa-resource-name>)  [unwired: 1 in, 2 out]
                }
                frame #13 {
                  n149 = Wait (ms)(milliseconds to wait=u32 5) -> ()  [unwired: 1 out]
                }
                frame #14 {
                  n150 = Greater?(x=w219, y=w218) -> (0:w220:bool)
                  n151 = case shown="True" w220 {
                    tunnel: ["-1" "1"] -> w221
                    frame False {
                    }
                    frame True {
                    }
                  }
                  n152 = Concatenate Strings(":SOUR:VOLT:STEP " ("write buffer 2"), w221) -> (w223:string)
                  n153 = VISA Write(VISA resource name=w225, write buffer=w223) -> (VISA resource name out=w224:refnum<visa-resource-name>)  [unwired: 1 in, 2 out]
                }
                frame #15 {
                  n154 = Wait (ms)(milliseconds to wait=u32 5) -> ()  [unwired: 1 out]
                }
                frame #16 {
                  n155 = Subtract(x=w240, y=w239) -> (x-y=w238:dbl)
                  n156 = Absolute Value(x=w238) -> (abs(x)=w234:dbl)
                  n157 = Add(x=w234, y=1) -> (x+y=w232:dbl)
                  n158 = Number To Fractional String(number=w232) -> (F-format string=w236:string)  [unwired: 3 in]
                  n159 = Concatenate Strings(":TRIG:COUN " ("write buffer 2"), w236) -> (w237:string)
                  n160 = VISA Write(VISA resource name=w242, write buffer=w237) -> (VISA resource name out=w241:refnum<visa-resource-name>)  [unwired: 1 in, 2 out]
                }
                frame #17 {
                  n161 = Wait (ms)(milliseconds to wait=u32 5) -> ()  [unwired: 1 out]
                }
                frame #18 {
                  n162 = VISA Write(VISA resource name=w246, write buffer=":OUTP ON" ("write buffer 2")) -> (VISA resource name out=w245:refnum<visa-resource-name>)  [unwired: 1 in, 2 out]
                }
                frame #19 {
                  n163 = Wait (ms)(milliseconds to wait=u32 5) -> ()  [unwired: 1 out]
                }
                frame #20 {
                  n164 = VISA Write(VISA resource name=w251, write buffer=":READ?" ("write buffer 2")) -> (VISA resource name out=w250:refnum<visa-resource-name>)  [unwired: 1 in, 2 out]
                }
                frame #21 {
                  n165 = Wait (ms)(milliseconds to wait=u32 5) -> ()  [unwired: 1 out]
                }
                frame #22 {
                  n166 = VISA Read(VISA resource name=w257, byte count=u32 100) -> (read buffer=→"read buffer":string)  [unwired: 1 in, 3 out]
                }
                frame #23 {
                  n167 = local write "Apply voltage"(FALSE) -> ()
                }
              }
            }
          }
          n168 = case shown="False" "Set Temperature" {
            tunnel: w56 -> [w282 w337]
            tunnel: [w280 w334] -> w42
            tunnel: w37 -> [w281 w334]
            tunnel: w53 -> [w279 _]
            tunnel: [w278 w333] -> w40
            tunnel: w52 -> [w277 w333]
            tunnel: [w273 0.0] -> w50
            frame False {
              n169 = flat-sequence {
                tunnel: w282 -> [w298]
                tunnel: [w297] -> w272
                tunnel: w272 -> [w300]
                tunnel: [w300] -> w271
                tunnel: [w302] -> w274
                tunnel: [w305] -> w273
                tunnel: w271 -> [w304]
                tunnel: [w306] -> w270
                tunnel: w274 -> [w306]
                tunnel: w270 -> [w312]
                tunnel: [w311] -> w269
                tunnel: w269 -> [w314]
                tunnel: [w314] -> w268
                tunnel: w268 -> [w315]
                tunnel: [w316] -> w275
                tunnel: w275 -> [w321]
                frame #0 {
                  n170 = Concatenate Strings("KRDG? B" ("write buffer"), "\n") -> (w294:string)
                  n171 = VISA Write(VISA resource name=w298, write buffer=w294) -> (VISA resource name out=w297:refnum<visa-resource-name>)  [unwired: 1 in, 2 out]
                }
                frame #1 {
                  n172 = Wait (ms)(milliseconds to wait=5) -> ()  [unwired: 1 out]
                }
                frame #2 {
                  n173 = VISA Read(VISA resource name=w304, byte count=u32 100) -> (VISA resource name out=w302:refnum<visa-resource-name>, read buffer=w303:string)  [unwired: 1 in, 2 out]
                  n174 = Fract/Exp String To Number(string=w303) -> (number=w305:dbl)  [unwired: 3 in, 1 out]
                  "Sample Temp [K]" <- w305
                }
                frame #3 {
                  n175 = Wait (ms)(milliseconds to wait=5) -> ()  [unwired: 1 out]
                }
                frame #4 {
                  n176 = Concatenate Strings("KRDG? A" ("write buffer"), "\n") -> (w308:string)
                  n177 = VISA Write(VISA resource name=w312, write buffer=w308) -> (VISA resource name out=w311:refnum<visa-resource-name>)  [unwired: 1 in, 2 out]
                }
                frame #5 {
                  n178 = Wait (ms)(milliseconds to wait=10) -> ()  [unwired: 1 out]
                }
                frame #6 {
                  n179 = VISA Read(VISA resource name=w315, byte count=u32 100) -> (VISA resource name out=w316:refnum<visa-resource-name>, read buffer=w318:string)  [unwired: 1 in, 2 out]
                  n180 = Fract/Exp String To Number(string=w318) -> (number=→"VTI [K]":dbl)  [unwired: 3 in, 1 out]
                }
                frame #7 {
                  n181 = case shown="True" "Set VTI Heater Range" {
                    tunnel: w321 -> [_ w322]
                    frame False {
                    }
                    frame True {
                      n182 = flat-sequence {
                        tunnel: w322 -> [w325]
                        frame #0 {
                          n183 = Number To Fractional String(number="0:OFF\n1:2.5mW\n2:25mW\n3:250mW\n4:2.5W\n5:25W") -> (F-format string=w323:string)  [unwired: 3 in]
                          n184 = Concatenate Strings("RANGE " ("write buffer"), w323, "\n") -> (w326:string)
                          n185 = VISA Write(VISA resource name=w325, write buffer=w326) -> ()  [unwired: 1 in, 3 out]
                        }
                        frame #1 {
                          n186 = local write "Set VTI Heater Range"(FALSE) -> ()
                        }
                      }
                    }
                  }
                }
              }
              n187 = case shown="False" "Reset" {
                tunnel: w273 -> [w288 _]
                tunnel: w281 -> [w287 _]
                tunnel: [w286 w290] -> w280
                tunnel: w279 -> [w285 _]
                tunnel: [w284 w289] -> w278
                tunnel: w277 -> [w283 _]
                frame False {
                  n188 = Build Array (concatenate)(w287, w288) -> (w286:dbl[])
                  n189 = Build Array (concatenate)(w283, w285) -> (w284:dbl[])
                }
                frame True {
                  n190 = stacked-sequence {
                    tunnel: [dbl[] [] _] -> w290
                    tunnel: [dbl[] [] _] -> w289
                    frame #0 {
                    }
                    frame #1 {
                      n191 = local write "Reset"(FALSE) -> ()
                    }
                  }
                }
              }
            }
            frame True {
              n192 = Number To Fractional String(number="1:VTI 2:Sample") -> (F-format string=w330:string)  [unwired: 3 in]
              n193 = stacked-sequence {
                tunnel: w337 -> [w338 _ w348 _ w358 _]
                tunnel: "Set Temp [K]" -> [_ _ _ _ w357 _]
                tunnel: "Rate [K/min]" -> [_ _ w347 _ _ _]
                tunnel: w330 -> [_ _ w343 _ w352 _]
                frame #0 {
                  n194 = Concatenate Strings("OUTMODE 1, 1, 2, 1" ("write buffer"), "\n") -> (w339:string)
                  n195 = VISA Write(VISA resource name=w338, write buffer=w339) -> ()  [unwired: 1 in, 3 out]
                }
                frame #1 {
                  n196 = Wait (ms)(milliseconds to wait=u32 50) -> ()  [unwired: 1 out]
                }
                frame #2 {
                  n197 = Number To Fractional String(number=w347) -> (F-format string=w345:string)  [unwired: 3 in]
                  n198 = Concatenate Strings("RAMP " ("write buffer"), w343, ", 1," ("write buffer"), w345, "\n") -> (w350:string)
                  n199 = VISA Write(VISA resource name=w348, write buffer=w350) -> ()  [unwired: 1 in, 3 out]
                }
                frame #3 {
                  n200 = Wait (ms)(milliseconds to wait=u32 50) -> ()  [unwired: 1 out]
                }
                frame #4 {
                  n201 = Number To Fractional String(number=w357) -> (F-format string=w355:string)  [unwired: 3 in]
                  n202 = Concatenate Strings("SETP " ("write buffer"), w352, "," ("write buffer"), w355, "\n") -> (w359:string)
                  n203 = VISA Write(VISA resource name=w358, write buffer=w359) -> ()  [unwired: 1 in, 3 out]
                }
                frame #5 {
                  n204 = local write "Set Temperature"(FALSE) -> ()
                }
              }
            }
          }
          n205 = Get Date/Time In Seconds() -> (seconds since 1Jan1904=w34:timestamp)
          n206 = Subtract(x=w33, y=w34) -> (x-y=w49:dbl)
          n207 = Subtract(x=w51, y=w50) -> (x-y=w46:dbl)
          n208 = call "Convert to Dynamic Data7"("Array"=w42) -> ("Dynamic Data Type"=w45:dynamicdata)  [unwired: 3 in]
          n209 = call "Convert to Dynamic Data9"("Array"=w42) -> ("Dynamic Data Type"=w41:dynamicdata)  [unwired: 3 in]
          n210 = call "Convert to Dynamic Data8"("Array"=w40) -> ("Dynamic Data Type"=w44:dynamicdata)  [unwired: 3 in]
          n211 = call "Convert to Dynamic Data10"("Array"=w40) -> ("Dynamic Data Type"=w39:dynamicdata)  [unwired: 3 in]
          n212 = Divide(x=w49, y=60) -> (x/y=w47:dbl)
          n213 = Divide(x=w46, y=w47) -> (x/y=w31:dbl)
          n214 = case shown="True" "Measure R-T" {
            tunnel: w45 -> [_ w263]
            tunnel: w44 -> [_ w262]
            frame False {
            }
            frame True {
              n215 = call "Build XY Graph2"("Y Input"=w262, "X Input"=w263) -> ("XY Graph"=→"R-T":cluster{"X":dbl[], "Y":dbl[]}[])  [unwired: 8 in, 1 out]
              n216 = call "Time Delay16"("Delay Time (s)"="Period [s]") -> ()  [unwired: 10 in, 1 out]
            }
          }
          n217 = Merge Signals(w41, w39) -> (w43:dynamicdata)
          n218 = call <vilib>:"Mean PtByPt.vi"("x"=w31, "sample length"=3) -> ("mean"=→"Rate [K/min]":dbl)  [unwired: 2 in, 1 out]
          n219 = case shown="False" "Save R-T" {
            tunnel: w43 -> [_ w264]
            frame False {
            }
            frame True {
              n220 = flat-sequence {
                tunnel: w264 -> [w265]
                frame #0 {
                  n221 = call "Write To Measurement File2"("Signals"=w265, "Reset"=TRUE) -> ()  [unwired: 15 in, 3 out]
                }
                frame #1 {
                  n222 = local write "Save R-T"(FALSE) -> ()
                }
              }
            }
          }
          n223 = case shown="True" "Measure R-H" {
            frame False {
            }
            frame True {
              n224 = local write "Measure R-T"(FALSE) -> ()
            }
          }
        }
      }
      frame #1 {
        # "interlocks"
        n225 = while {
          tunnel: "Set Temp [K]  Rate [K/min]" -> [w568]
          tunnel: w534 -> [w566]
          tunnel: w533 -> [w565]
          tunnel: w532 -> [w564]
          tunnel: w530 -> [w555]
          tunnel: w529 -> [w554]
          tunnel: w528 -> [w553]
          tunnel: w527 -> [w552]
          i -> [w567]
          stop <- w556 stop-if-true
          n226 = Matrix Size(0:w568) -> (1:w569:i32)  [unwired: 1 out]
          n227 = Less Or Equal?(x=w569, y=w567) -> (x <= y?=w559:bool)
          n228 = Index Array(array=w568, index (row)=w567) -> (element=w570:dbl[])  [unwired: 1 in]
          n229 = Index Array(array=w570, index=1) -> (element=w562:dbl)
          n230 = Index Array(array=w570, index=0) -> (element=w561:dbl)
          n231 = Multiply(x=w562, y=w561) -> (x*y=w563:dbl)
          n232 = Equal To 0?(x=w563) -> (x = 0?=w560:bool)
          n233 = Or(x=w560, y=w559) -> (x .or. y?=w558:bool)
          n234 = case shown="False" w558 {
            tunnel: w566 -> [w583 _]
            tunnel: w562 -> [w582 _]
            tunnel: w565 -> [w576 _]
            tunnel: w564 -> [w581 _]
            tunnel: w561 -> [w580 _]
            tunnel: [w579 FALSE ("Boolean")] -> w557
            tunnel: w555 -> [w577 _]
            tunnel: w554 -> [w575 _]
            tunnel: w553 -> [w574 _]
            tunnel: w552 -> [w573 _]
            frame False {
              n235 = stacked-sequence {
                tunnel: w583 -> [w584 w700]
                tunnel: w580 -> [w589 _]
                tunnel: w582 -> [w588 _]
                tunnel: w576 -> [w587 w699]
                tunnel: w581 -> [_ w698]
                tunnel: w580 -> [_ w697]
                tunnel: [_ w696] -> w579
                tunnel: "Field [T]" -> [w586 w695]
                tunnel: w577 -> [w585 _]
                tunnel: w575 -> [_ w694]
                tunnel: w574 -> [_ w693]
                tunnel: w573 -> [_ w692]
                frame #0 {
                  n236 = flat-sequence {
                    tunnel: w585 -> [w594]
                    tunnel: w589 -> [w593]
                    tunnel: w588 -> [w592]
                    tunnel: w584 -> [w590]
                    tunnel: w587 -> [w656]
                    tunnel: w586 -> [w654]
                    frame #0 {
                      n237 = case shown="False" "Temp control off" {
                        tunnel: w594 -> [w597 _]
                        tunnel: w593 -> [w600 _]
                        tunnel: w592 -> [w599 _]
                        tunnel: w590 -> [w595 _]
                        frame False {
                          n238 = case shown="False" "Main sorb T control" {
                            tunnel: w597 -> [_ w602]
                            tunnel: [w601 w602] -> w596
                            tunnel: w595 -> [w601 _]
                            frame False {
                            }
                            frame True {
                            }
                          }
                          n239 = stacked-sequence {
                            tunnel: w596 -> [w603 _ w613 _ w623 w627]
                            tunnel: w600 -> [_ _ _ _ w622 _]
                            tunnel: w599 -> [_ _ w614 _ _ _]
                            tunnel: "Main sorb T control" -> [w604 _ _ _ _ w628]
                            frame #0 {
                              n240 = case shown="False" w604 {
                                tunnel: ["OUTMODE 1, 1, 2, 1" ("write buffer") "OUTMODE1,1,1,1" ("write buffer")] -> w605
                                frame False {
                                }
                                frame True {
                                }
                              }
                              n241 = Concatenate Strings(w605, "\n") -> (w606:string)
                              n242 = VISA Write(VISA resource name=w603, write buffer=w606) -> ()  [unwired: 1 in, 3 out]
                            }
                            frame #1 {
                              n243 = Wait (ms)(milliseconds to wait=u32 50) -> ()  [unwired: 1 out]
                            }
                            frame #2 {
                              n244 = case shown="False" "T-ramp off" {
                                tunnel: ["RAMP 1, 1," ("write buffer") "RAMP 1, 0," ("write buffer")] -> w612
                                frame False {
                                }
                                frame True {
                                }
                              }
                              n245 = Number To Fractional String(number=w614) -> (F-format string=w615:string)  [unwired: 3 in]
                              n246 = Concatenate Strings(w612, w615, "\n") -> (w616:string)
                              n247 = VISA Write(VISA resource name=w613, write buffer=w616) -> ()  [unwired: 1 in, 3 out]
                            }
                            frame #3 {
                              n248 = Wait (ms)(milliseconds to wait=u32 50) -> ()  [unwired: 1 out]
                            }
                            frame #4 {
                              n249 = Number To Fractional String(number=w622) -> (F-format string=w621:string)  [unwired: 3 in]
                              n250 = Concatenate Strings("SETP 1," ("write buffer"), w621, "\n") -> (w625:string)
                              n251 = VISA Write(VISA resource name=w623, write buffer=w625) -> ()  [unwired: 1 in, 3 out]
                            }
                            frame #5 {
                              n252 = flat-sequence {
                                tunnel: w628 -> [w630]
                                tunnel: w627 -> [w629]
                                frame #0 {
                                n253 = while {
                                tunnel: w630 -> [w633]
                                tunnel: w629 -> [w632]
                                i -> [w631]
                                stop <- w645 stop-if-true
                                n254 = case shown="False" w633 {
                                tunnel: ["KRDG? B" ("write buffer") "KRDG? A" ("write buffer")] -> w634
                                frame False {
                                }
                                frame True {
                                }
                                }
                                n255 = Wait (ms)(milliseconds to wait=1000) -> ()  [unwired: 1 out]
                                n256 = Multiply(x="Wait T-stable [min]", y=60) -> (x*y=w644:i32)
                                n257 = Concatenate Strings(w634, "\n") -> (w639:string)
                                n258 = Less?(x=w644, y=w631) -> (x < y?=w643:bool)
                                n259 = VISA Write(VISA resource name=w632, write buffer=w639) -> (VISA resource name out=w638:refnum<visa-resource-name>)  [unwired: 1 in, 2 out]
                                n260 = Or(x=w643, y="Skip") -> (x .or. y?=w645:bool)
                                n261 = VISA Read(VISA resource name=w638, byte count=u32 100) -> (read buffer=w636:string)  [unwired: 1 in, 3 out]
                                n262 = Fract/Exp String To Number(string=w636) -> (number=→"temp [K]":dbl)  [unwired: 3 in, 1 out]
                                "Waiting T-stability" <- TRUE
                                }
                                }
                                frame #1 {
                                w651 = FALSE
                                n263 = local write "Reset"(TRUE) -> ()
                                n264 = local write "Skip"(w651) -> ()
                                n265 = local write "Waiting T-stability"(w651) -> ()
                                }
                              }
                            }
                          }
                        }
                        frame True {
                          n266 = local write "Reset"(TRUE) -> ()
                        }
                      }
                    }
                    frame #1 {
                      n267 = case shown="True" "Set Initial Field" {
                        tunnel: w656 -> [_ w659]
                        tunnel: w654 -> [_ w657]
                        frame False {
                        }
                        frame True {
                          n268 = stacked-sequence {
                            tunnel: w659 -> [w660 w663 _ w681 _ w686 _]
                            tunnel: 0.2 -> [_ _ _ w671 _ _ _]
                            tunnel: w657 -> [_ w661 _ _ _ _ _]
                            frame #0 {
                              n269 = VISA Clear(VISA resource name=w660) -> ()  [unwired: 1 in, 2 out]
                            }
                            frame #1 {
                              # "set set field"
                              n270 = Number To Fractional String(number=w661, width (-)=i16 6, precision (6)=i16 3) -> (F-format string=w666:string)  [unwired: 1 in]
                              n271 = Concatenate Strings("S [%][MID] " ("string"), w666) -> (w662:string)
                              n272 = Concatenate Strings(w662, "\r") -> (w665:string)
                              n273 = VISA Write(VISA resource name=w663, write buffer=w665) -> ()  [unwired: 1 in, 3 out]
                            }
                            frame #2 {
                              n274 = Wait (ms)(milliseconds to wait=500) -> ()  [unwired: 1 out]
                            }
                            frame #3 {
                              # "set rate"
                              n275 = Divide(x=w671, y=60.0) -> (x/y=w676:dbl)
                              n276 = Divide(x=w676, y=0.09797) -> (x/y=w674:dbl)
                              n277 = Number To Fractional String(number=w674, width (-)=i16 6, precision (6)=i16 3) -> (F-format string=w679:string)  [unwired: 1 in]
                              n278 = Concatenate Strings("S R " ("string"), w679) -> (w678:string)
                              n279 = Concatenate Strings(w678, "\r") -> (w683:string)
                              n280 = VISA Write(VISA resource name=w681, write buffer=w683) -> ()  [unwired: 1 in, 3 out]
                            }
                            frame #4 {
                              n281 = Wait (ms)(milliseconds to wait=500) -> ()  [unwired: 1 out]
                            }
                            frame #5 {
                              # "Go to set field"
                              n282 = Concatenate Strings("R [%][MID]" ("data"), "\r") -> (w688:string)
                              n283 = VISA Write(VISA resource name=w686, write buffer=w688) -> ()  [unwired: 1 in, 3 out]
                            }
                            frame #6 {
                              n284 = Multiply(x="Wait [min]", y=60000) -> (x*y=w691:i32)
                              n285 = Wait (ms)(milliseconds to wait=w691) -> ()  [unwired: 1 out]
                            }
                          }
                        }
                      }
                    }
                  }
                }
                frame #1 {
                  n286 = flat-sequence {
                    tunnel: [w716] -> w707
                    tunnel: [w717] -> w706
                    tunnel: ["Set Field [T]   Rate [T/min]"] -> w705
                    tunnel: w699 -> [w717]
                    tunnel: w698 -> [w716]
                    tunnel: w695 -> [w713]
                    tunnel: w707 -> [w741]
                    tunnel: [w741] -> w704
                    tunnel: [w740] -> w703
                    tunnel: w706 -> [w740]
                    tunnel: [w740] -> w702
                    tunnel: [w739] -> w701
                    tunnel: w705 -> [w739]
                    tunnel: w704 -> [w751]
                    tunnel: w703 -> [w750]
                    tunnel: w702 -> [w749]
                    tunnel: w701 -> [w748]
                    tunnel: w700 -> [w747]
                    tunnel: w697 -> [w746]
                    tunnel: [w745] -> w696
                    tunnel: w694 -> [w744]
                    tunnel: w693 -> [w743]
                    tunnel: w692 -> [w742]
                    frame #0 {
                      # "interlocks"
                      n287 = Greater?(x=w713, y=10) -> (0:w712:bool)
                      n288 = Less?(x=w713, y=-10) -> (x < y?=w711:bool)
                      n289 = Or(x=w712, y=w711) -> (x .or. y?=w710:bool)
                      n290 = Index Array(array="Set Field [T]   Rate [T/min]", index (col)=0) -> (element=w725:dbl[])  [unwired: 1 in]
                      n291 = Array Max & Min(array=w725) -> (max value=w718:dbl, min value=w728:dbl)  [unwired: 2 out]
                      n292 = Index Array(array="Set Field [T]   Rate [T/min]", index (col)=1) -> (element=w736:dbl[])  [unwired: 1 in]
                      n293 = Array Max & Min(array=w736) -> (max value=w730:dbl, min value=w733:dbl)  [unwired: 2 out]
                      n294 = Greater?(x=w718, y=10) -> (0:w719:bool)
                      n295 = Less?(x=w728, y=-10) -> (x < y?=w729:bool)
                      n296 = Or(x=w719, y=w729) -> (x .or. y?=w709:bool)
                      n297 = Greater?(x=w730, y=0.6) -> (0:w735:bool)
                      n298 = Less?(x=w733, y=-0.6) -> (x < y?=w734:bool)
                      n299 = Or(x=w710, y=w709) -> (x .or. y?=w708:bool)
                      n300 = Or(x=w735, y=w734) -> (x .or. y?=w737:bool)
                      n301 = call "Display Message to User4"("Enable"=w708) -> ("OK"=w738:bool)  [unwired: 9 in, 1 out]
                      n302 = call "Display Message to User3"("Enable"=w737) -> ("OK"=w720:bool)  [unwired: 9 in, 1 out]
                      n303 = Or(x=w738, y=w720) -> (x .or. y?=w721:bool)
                      n304 = Stop(stop? (T)=w721) -> ()
                    }
                    frame #1 {
                    }
                    frame #2 {
                      n305 = while {
                        tunnel: w751 -> [w772]
                        tunnel: w750 -> [w771]
                        tunnel: w749 -> [w766]
                        tunnel: w748 -> [w763]
                        tunnel: w747 -> [w762]
                        tunnel: w746 -> [w761]
                        tunnel: [w755] -> w745
                        tunnel: w744 -> [w754]
                        tunnel: w743 -> [w753]
                        tunnel: w742 -> [w752]
                        i -> [w767]
                        stop <- w756 stop-if-true
                        n306 = Matrix Size(0:w763) -> (1:w764:i32)  [unwired: 1 out]
                        n307 = Less Or Equal?(x=w764, y=w767) -> (x <= y?=w758:bool)
                        n308 = Index Array(array=w763, index (row)=w767) -> (element=w768:dbl[])  [unwired: 1 in]
                        n309 = Index Array(array=w768, index=1) -> (element=w760:dbl)
                        n310 = Index Array(array=w768, index=0) -> (element=w765:dbl)
                        n311 = Equal To 0?(x=w760) -> (x = 0?=w759:bool)
                        n312 = Or(x=w759, y=w758) -> (x .or. y?=w757:bool)
                        n313 = case shown="False" w757 {
                          tunnel: w772 -> [w783 _]
                          tunnel: w771 -> [w782 _]
                          tunnel: w760 -> [w781 _]
                          tunnel: w766 -> [w780 _]
                          tunnel: w765 -> [w779 _]
                          tunnel: w762 -> [w778 _]
                          tunnel: w761 -> [w777 _]
                          tunnel: [w776 FALSE] -> w755
                          tunnel: w754 -> [w775 _]
                          tunnel: w753 -> [w774 _]
                          tunnel: w752 -> [w773 _]
                          frame False {
                            n314 = stacked-sequence {
                              tunnel: w783 -> [_ w870]
                              tunnel: w782 -> [_ w869]
                              tunnel: w780 -> [w786 _]
                              tunnel: w779 -> [w785 w868]
                              tunnel: w781 -> [w784 _]
                              tunnel: w778 -> [_ w867]
                              tunnel: w777 -> [_ w866]
                              tunnel: [_ w865] -> w776
                              tunnel: w775 -> [_ w864]
                              tunnel: w774 -> [_ w863]
                              tunnel: w773 -> [_ w862]
                              frame #0 {
                                n315 = stacked-sequence {
                                tunnel: w785 -> [_ _ w794 _ w837 _ _ _ _ _]
                                tunnel: w786 -> [w787 _ w790 _ w834 _ w853 _ w858 _]
                                tunnel: w784 -> [_ _ _ _ _ _ w846 _ _ _]
                                frame #0 {
                                n316 = VISA Clear(VISA resource name=w787) -> ()  [unwired: 1 in, 2 out]
                                }
                                frame #1 {
                                n317 = Wait (ms)(milliseconds to wait=500) -> ()  [unwired: 1 out]
                                }
                                frame #2 {
                                # "Read Magnetic Field"
                                # "for safety"
                                # "polarity"
                                n318 = stacked-sequence {
                                seq-local: [w795 _ _ _ _ _ _ _] -> [_ w798 _ _ _ _ _ _]
                                seq-local: [_ w796 _ _ _ _ _ _] -> [_ _ w800 _ _ _ _ _]
                                seq-local: [_ w797 _ _ _ _ _ _] -> [_ _ w799 _ _ _ _ _]
                                seq-local: [_ _ w800 _ _ _ _ _] -> [_ _ _ w803 _ _ _ _]
                                seq-local: [_ _ w799 _ _ _ _ _] -> [_ _ _ w802 _ _ _ _]
                                seq-local: [_ _ _ w805 _ _ _ _] -> [_ _ _ _ w808 _ _ _]
                                seq-local: [_ _ _ w804 _ _ _ _] -> [_ _ _ _ w809 _ _ _]
                                seq-local: [_ _ _ _ w808 _ _ _] -> [_ _ _ _ _ w820 _ _]
                                seq-local: [_ _ _ _ w809 _ _ _] -> [_ _ _ _ _ w818 _ _]
                                seq-local: [_ _ _ _ _ w819 _ _] -> [_ _ _ _ _ _ _ w823]
                                seq-local: [_ _ _ _ _ w817 _ _] -> [_ _ _ _ _ _ _ w822]
                                tunnel: w790 -> [w795 _ _ _ _ _ _ _]
                                tunnel: [_ _ _ _ _ w810 _ _] -> w791
                                frame #0 {
                                }
                                frame #1 {
                                n319 = VISA Clear(VISA resource name=w798) -> (VISA resource name out=w796:refnum<visa-resource-name>, error out=w797:errorcluster)  [unwired: 1 in]
                                }
                                frame #2 {
                                n320 = call "Time Delay4"() -> ()  [unwired: 11 in, 1 out]
                                }
                                frame #3 {
                                n321 = Concatenate Strings("G O" ("Command"), "\r") -> (w806:string)
                                n322 = VISA Write(VISA resource name=w803, write buffer=w806, error in (no error)=w802) -> (VISA resource name out=w805:refnum<visa-resource-name>, error out=w804:errorcluster)  [unwired: 1 out]
                                }
                                frame #4 {
                                n323 = call "Time Delay5"() -> ()  [unwired: 11 in, 1 out]
                                }
                                frame #5 {
                                n324 = VISA Read(VISA resource name=w820, byte count=u32 30, error in (no error)=w818) -> (VISA resource name out=w819:refnum<visa-resource-name>, read buffer=w814:string, error out=w817:errorcluster)  [unwired: 1 out]
                                n325 = Match Pattern(string=w814, regular expression="OUTPUT:") -> (after substring=w812:string)  [unwired: 1 in, 3 out]
                                n326 = Match Pattern(string=w812, regular expression=" TESLA") -> (before substring=w811:string)  [unwired: 1 in, 3 out]
                                n327 = Fract/Exp String To Number(string=w811, offset=0) -> (number=w810:dbl)  [unwired: 2 in, 1 out]
                                }
                                frame #6 {
                                n328 = call "Time Delay13"() -> ()  [unwired: 11 in, 1 out]
                                }
                                frame #7 {
                                n329 = VISA Close(VISA resource name=w823, error in (no error)=w822) -> ()  [unwired: 1 out]
                                }
                                }
                                n330 = Absolute Value(x=w791) -> (abs(x)=w792:dbl)
                                n331 = Less?(x=w792, y=0.05) -> (x < y?=w789:bool)
                                n332 = case shown="False" w789 {
                                tunnel: w794 -> [_ w825]
                                tunnel: w790 -> [_ w826]
                                frame False {
                                }
                                frame True {
                                n333 = Greater Or Equal To 0?(x=w825) -> (x >= 0?=w824:bool)
                                n334 = case shown="True" w824 {
                                tunnel: ["D [-]" ("data") "D [+]" ("data")] -> w827
                                frame False {
                                }
                                frame True {
                                }
                                }
                                n335 = Concatenate Strings(w827, "\r") -> (w829:string)
                                n336 = VISA Write(VISA resource name=w826, write buffer=w829) -> ()  [unwired: 1 in, 3 out]
                                }
                                }
                                }
                                frame #3 {
                                n337 = Wait (ms)(milliseconds to wait=500) -> ()  [unwired: 1 out]
                                }
                                frame #4 {
                                # "set set field"
                                n338 = Number To Fractional String(number=w837, width (-)=i16 6, precision (6)=i16 3) -> (F-format string=w838:string)  [unwired: 1 in]
                                n339 = Concatenate Strings("S [%][MID] " ("string"), w838) -> (w833:string)
                                n340 = Concatenate Strings(w833, "\r") -> (w836:string)
                                n341 = VISA Write(VISA resource name=w834, write buffer=w836) -> ()  [unwired: 1 in, 3 out]
                                }
                                frame #5 {
                                n342 = Wait (ms)(milliseconds to wait=500) -> ()  [unwired: 1 out]
                                }
                                frame #6 {
                                # "set rate"
                                n343 = Divide(x=w846, y=60.0) -> (x/y=w848:dbl)
                                n344 = Divide(x=w848, y=0.09797) -> (x/y=w843:dbl)
                                n345 = Number To Fractional String(number=w843, width (-)=i16 6, precision (6)=i16 3) -> (F-format string=w851:string)  [unwired: 1 in]
                                n346 = Concatenate Strings("S R " ("string"), w851) -> (w850:string)
                                n347 = Concatenate Strings(w850, "\r") -> (w855:string)
                                n348 = VISA Write(VISA resource name=w853, write buffer=w855) -> ()  [unwired: 1 in, 3 out]
                                }
                                frame #7 {
                                n349 = Wait (ms)(milliseconds to wait=500) -> ()  [unwired: 1 out]
                                }
                                frame #8 {
                                # "Go to set field"
                                n350 = Concatenate Strings("R [%][MID]" ("data"), "\r") -> (w860:string)
                                n351 = VISA Write(VISA resource name=w858, write buffer=w860) -> ()  [unwired: 1 in, 3 out]
                                }
                                frame #9 {
                                n352 = Wait (ms)(milliseconds to wait=500) -> ()  [unwired: 1 out]
                                }
                                }
                              }
                              frame #1 {
                                n353 = while {
                                tunnel: w870 -> [w893]
                                tunnel: w869 -> [w894]
                                tunnel: w868 -> [w892]
                                tunnel: w867 -> [w890]
                                tunnel: w866 -> [w889]
                                shift-right: [w881] -> _
                                shift-left: _ -> [w888]
                                shift-right: [w884] -> _
                                shift-left: _ -> [w887]
                                shift-right: [w883] -> _
                                shift-left: _ -> [w886]
                                shift-right: [w882] -> _
                                shift-left: _ -> [w885]
                                tunnel: ["Stop"] -> w865
                                tunnel: w864 -> [w877]
                                tunnel: w863 -> [w876]
                                shift-right: [w875] -> _
                                shift-left: _ -> [w874]
                                shift-right: [w873] -> _
                                shift-left: _ -> [w872]
                                tunnel: w862 -> [w871]
                                stop <- w880 stop-if-true
                                n354 = while {
                                stop <- "stop 2" continue-if-true
                                }
                                n355 = stacked-sequence {
                                seq-local: [w903 _ _ _ _ _] -> [_ w968 _ _ _ _]
                                seq-local: [w902 _ _ _ _ _] -> [_ w967 _ _ _ _]
                                seq-local: [_ w969 _ _ _ _] -> [_ _ w989 _ _ _]
                                seq-local: [_ w959 _ _ _ _] -> [_ _ w988 _ _ _]
                                seq-local: [_ w967 _ _ _ _] -> [_ _ w980 _ _ _]
                                seq-local: [_ w958 _ _ _ _] -> [_ _ w978 _ _ _]
                                seq-local: [_ _ w989 _ _ _] -> [_ _ _ w1032 _ _]
                                seq-local: [_ _ w988 _ _ _] -> [_ _ _ w1031 _ _]
                                seq-local: [_ _ w979 _ _ _] -> [_ _ _ w1030 _ _]
                                seq-local: [_ _ w978 _ _ _] -> [_ _ _ w1023 _ _]
                                seq-local: [_ _ _ w1032 _ _] -> [_ _ _ _ w1097 _]
                                seq-local: [_ _ _ w1031 _ _] -> [_ _ _ _ w1090 _]
                                seq-local: [_ _ _ w1030 _ _] -> [_ _ _ _ w1091 _]
                                seq-local: [_ _ _ w1030 _ _] -> [_ _ _ _ _ _]
                                seq-local: [_ _ _ w1022 _ _] -> [_ _ _ _ w1087 _]
                                seq-local: [w896 _ _ _ _ _] -> [_ _ _ _ w1034 _]
                                seq-local: [w899 _ _ _ _ _] -> [_ _ _ _ w1033 _]
                                tunnel: w893 -> [w904 _ _ _ _ _]
                                tunnel: w894 -> [w902 _ _ _ _ _]
                                tunnel: w890 -> [_ w960 _ _ _ _]
                                tunnel: w892 -> [_ _ w987 _ _ _]
                                tunnel: [_ _ w985 _ _ _] -> w891
                                tunnel: [_ _ _ _ w1097 _] -> _
                                tunnel: w889 -> [_ _ _ _ w1093 _]
                                tunnel: [_ _ _ _ w1074 _] -> w881
                                tunnel: w888 -> [_ _ _ _ w1086 _]
                                tunnel: [_ _ _ _ w1068 _] -> w884
                                tunnel: w887 -> [_ _ _ _ w1081 _]
                                tunnel: [_ _ _ _ w1070 _] -> w883
                                tunnel: w886 -> [_ _ _ _ w1040 _]
                                tunnel: [_ _ _ _ w1071 _] -> w882
                                tunnel: w885 -> [_ _ _ _ w1089 _]
                                tunnel: w877 -> [w901 w956 _ _ w1035 _]
                                tunnel: w876 -> [w900 _ _ _ _ _]
                                tunnel: [_ _ _ _ w1045 _] -> w875
                                tunnel: w874 -> [_ _ _ _ w1039 _]
                                tunnel: [_ _ _ _ w1043 _] -> w873
                                tunnel: w872 -> [_ _ _ _ w1038 _]
                                tunnel: w871 -> [w898 _ _ _ _ _]
                                frame #0 {
                                n356 = case shown="False" w901 {
                                tunnel: w904 -> [w909 w954]
                                tunnel: [w909 w953] -> w903
                                tunnel: w900 -> [w905 _]
                                tunnel: [w908 w952] -> w897
                                tunnel: [w907 w952] -> w899
                                frame False {
                                n357 = flat-sequence {
                                tunnel: [w914] -> w908
                                tunnel: w905 -> [w913]
                                tunnel: [w912] -> w906
                                tunnel: [w935] -> w907
                                tunnel: w906 -> [w934]
                                frame #0 {
                                n358 = flat-sequence {
                                tunnel: w913 -> [w918]
                                tunnel: [w917] -> w911
                                tunnel: w911 -> [w920]
                                tunnel: [w920] -> w910
                                tunnel: [w921] -> w916
                                tunnel: w910 -> [w923]
                                tunnel: [w924] -> w915
                                tunnel: w916 -> [w924]
                                tunnel: w915 -> [w929]
                                tunnel: [w927] -> w914
                                tunnel: [w926] -> w912
                                frame #0 {
                                n359 = VISA Clear(VISA resource name=w918) -> (VISA resource name out=w917:refnum<visa-resource-name>)  [unwired: 1 in, 1 out]
                                }
                                frame #1 {
                                n360 = Wait (ms)(milliseconds to wait=5) -> ()  [unwired: 1 out]
                                }
                                frame #2 {
                                n361 = VISA Write(VISA resource name=w923, write buffer="OUTP? 3" ("write buffer 2")) -> (VISA resource name out=w921:refnum<visa-resource-name>)  [unwired: 1 in, 2 out]
                                }
                                frame #3 {
                                n362 = Wait (ms)(milliseconds to wait=5) -> ()  [unwired: 1 out]
                                }
                                frame #4 {
                                n363 = VISA Read(VISA resource name=w929, byte count=u32 360) -> (VISA resource name out=w926:refnum<visa-resource-name>, read buffer=w928:string)  [unwired: 1 in, 2 out]
                                n364 = Fract/Exp String To Number(string=w928, offset=0) -> (number=w927:dbl)  [unwired: 3 out]
                                "Lockin x (V)" <- w927
                                }
                                }
                                }
                                frame #1 {
                                n365 = flat-sequence {
                                tunnel: w934 -> [w939]
                                tunnel: [w938] -> w933
                                tunnel: w933 -> [w941]
                                tunnel: [w941] -> w932
                                tunnel: [w942] -> w937
                                tunnel: w932 -> [w944]
                                tunnel: [w945] -> w936
                                tunnel: w937 -> [w945]
                                tunnel: w936 -> [w949]
                                tunnel: [w947] -> w935
                                frame #0 {
                                n366 = VISA Clear(VISA resource name=w939) -> (VISA resource name out=w938:refnum<visa-resource-name>)  [unwired: 1 in, 1 out]
                                }
                                frame #1 {
                                n367 = Wait (ms)(milliseconds to wait=5) -> ()  [unwired: 1 out]
                                }
                                frame #2 {
                                n368 = VISA Write(VISA resource name=w944, write buffer="OUTP? 4" ("write buffer 2")) -> (VISA resource name out=w942:refnum<visa-resource-name>)  [unwired: 1 in, 2 out]
                                }
                                frame #3 {
                                n369 = Wait (ms)(milliseconds to wait=5) -> ()  [unwired: 1 out]
                                }
                                frame #4 {
                                n370 = VISA Read(VISA resource name=w949, byte count=u32 360) -> (read buffer=w948:string)  [unwired: 1 in, 3 out]
                                n371 = Fract/Exp String To Number(string=w948, offset=0) -> (number=w947:dbl)  [unwired: 3 out]
                                "Lockin y (V)" <- w947
                                }
                                }
                                }
                                }
                                }
                                frame True {
                                w952 = 0.0
                                n372 = VISA Write(VISA resource name=w954, write buffer="SENS:DATA:LATest?") -> (VISA resource name out=w953:refnum<visa-resource-name>)  [unwired: 1 in, 2 out]
                                }
                                }
                                n373 = Divide(x=w897, y=w898) -> (x/y=w896:dbl)
                                }
                                frame #1 {
                                n374 = Concatenate Strings("KRDG? A" ("write buffer"), "\n") -> (w965:string)
                                n375 = VISA Write(VISA resource name=w960, write buffer=w965) -> (VISA resource name out=w963:refnum<visa-resource-name>)  [unwired: 1 in, 2 out]
                                n376 = VISA Read(VISA resource name=w963, byte count=u32 100) -> (VISA resource name out=w958:refnum<visa-resource-name>, read buffer=w961:string)  [unwired: 1 in, 2 out]
                                n377 = Fract/Exp String To Number(string=w961) -> (number=→"VTI [K]":dbl)  [unwired: 3 in, 1 out]
                                n378 = case shown="True" w956 {
                                tunnel: [w971 w977] -> w969
                                tunnel: w968 -> [w971 w973]
                                tunnel: [0.0 w972] -> w959
                                frame False {
                                }
                                frame True {
                                n379 = VISA Read(VISA resource name=w973, byte count=u32 360) -> (VISA resource name out=w977:refnum<visa-resource-name>, read buffer=w975:string)  [unwired: 1 in, 2 out]
                                n380 = Fract/Exp String To Number(string=w975, offset=0) -> (number=w972:dbl)  [unwired: 3 out]
                                }
                                }
                                "Delta reading [Ohm]" <- w959
                                }
                                frame #2 {
                                # "Read Magnetic Field"
                                n381 = stacked-sequence {
                                seq-local: [w990 _ _ _ _ _ _ _] -> [_ w993 _ _ _ _ _ _]
                                seq-local: [_ w991 _ _ _ _ _ _] -> [_ _ w995 _ _ _ _ _]
                                seq-local: [_ w992 _ _ _ _ _ _] -> [_ _ w994 _ _ _ _ _]
                                seq-local: [_ _ w995 _ _ _ _ _] -> [_ _ _ w998 _ _ _ _]
                                seq-local: [_ _ w994 _ _ _ _ _] -> [_ _ _ w997 _ _ _ _]
                                seq-local: [_ _ _ w1000 _ _ _ _] -> [_ _ _ _ w1003 _ _ _]
                                seq-local: [_ _ _ w999 _ _ _ _] -> [_ _ _ _ w1004 _ _ _]
                                seq-local: [_ _ _ _ w1003 _ _ _] -> [_ _ _ _ _ w1015 _ _]
                                seq-local: [_ _ _ _ w1004 _ _ _] -> [_ _ _ _ _ w1013 _ _]
                                seq-local: [_ _ _ _ _ w1014 _ _] -> [_ _ _ _ _ _ _ w1019]
                                seq-local: [_ _ _ _ _ w1012 _ _] -> [_ _ _ _ _ _ _ w1018]
                                tunnel: w980 -> [w990 _ _ _ _ _ _ _]
                                tunnel: [_ _ _ _ _ w1005 _ _] -> w979
                                frame #0 {
                                }
                                frame #1 {
                                n382 = VISA Clear(VISA resource name=w993) -> (VISA resource name out=w991:refnum<visa-resource-name>, error out=w992:errorcluster)  [unwired: 1 in]
                                }
                                frame #2 {
                                n383 = call "Time Delay2"() -> ()  [unwired: 11 in, 1 out]
                                }
                                frame #3 {
                                n384 = Concatenate Strings("G O" ("Command"), "\r") -> (w1001:string)
                                n385 = VISA Write(VISA resource name=w998, write buffer=w1001, error in (no error)=w997) -> (VISA resource name out=w1000:refnum<visa-resource-name>, error out=w999:errorcluster)  [unwired: 1 out]
                                }
                                frame #4 {
                                n386 = call "Time Delay3"() -> ()  [unwired: 11 in, 1 out]
                                }
                                frame #5 {
                                n387 = VISA Read(VISA resource name=w1015, byte count=u32 30, error in (no error)=w1013) -> (VISA resource name out=w1014:refnum<visa-resource-name>, read buffer=w1009:string, error out=w1012:errorcluster)  [unwired: 1 out]
                                n388 = Match Pattern(string=w1009, regular expression="OUTPUT:") -> (after substring=w1007:string)  [unwired: 1 in, 3 out]
                                n389 = Match Pattern(string=w1007, regular expression=" TESLA") -> (before substring=w1006:string)  [unwired: 1 in, 3 out]
                                n390 = Fract/Exp String To Number(string=w1006, offset=0) -> (number=w1005:dbl)  [unwired: 2 in, 1 out]
                                }
                                frame #6 {
                                n391 = call "Time Delay12"() -> ()  [unwired: 11 in, 1 out]
                                }
                                frame #7 {
                                n392 = VISA Close(VISA resource name=w1019, error in (no error)=w1018) -> (error out=→"error out 3":errorcluster)
                                }
                                }
                                "Magnetic Field [T]" <- w979
                                n393 = Equal To 0?(x=w979) -> (x = 0?=w982:bool)
                                n394 = case shown="False" w982 {
                                tunnel: w979 -> [w1020 _]
                                tunnel: [w1020 1.1] -> w981
                                frame False {
                                }
                                frame True {
                                }
                                }
                                n395 = Subtract(x=w981, y=w987) -> (x-y=w983:dbl)
                                n396 = Absolute Value(x=w983) -> (abs(x)=w984:dbl)
                                n397 = Less?(x=w984, y=0.03) -> (x < y?=w985:bool)
                                }
                                frame #3 {
                                n398 = Concatenate Strings("KRDG? B" ("write buffer"), "\n") -> (w1028:string)
                                n399 = VISA Write(VISA resource name=w1023, write buffer=w1028) -> (VISA resource name out=w1026:refnum<visa-resource-name>)  [unwired: 1 in, 2 out]
                                n400 = VISA Read(VISA resource name=w1026, byte count=u32 100) -> (read buffer=w1024:string)  [unwired: 1 in, 3 out]
                                n401 = Fract/Exp String To Number(string=w1024) -> (number=w1022:dbl)  [unwired: 3 in, 1 out]
                                "Sample Temp [K]" <- w1022
                                }
                                frame #4 {
                                # "Y(ohm)"
                                # "X(Ohm)"
                                # "Temp"
                                # "Delta"
                                # "Field"
                                # "Time"
                                n402 = case shown="False" w1035 {
                                tunnel: [w1109 w1110] -> w1041
                                tunnel: w1040 -> [_ w1110]
                                tunnel: w1038 -> [w1109 _]
                                frame False {
                                }
                                frame True {
                                }
                                }
                                n403 = call "Convert to Dynamic Data12"("Array"=w1039) -> ("Dynamic Data Type"=w1036:dynamicdata)  [unwired: 3 in]
                                n404 = call "Convert to Dynamic Data11"("Array"=w1038) -> ("Dynamic Data Type"=w1037:dynamicdata)  [unwired: 3 in]
                                n405 = call "Convert to Dynamic Data5"("Array"=w1081) -> ("Dynamic Data Type"=w1066:dynamicdata)  [unwired: 3 in]
                                n406 = Path To String(path="Folder") -> (string=w1077:string)
                                n407 = Number To Fractional String(number=w1093, precision (6)=2) -> (F-format string=w1094:string)  [unwired: 2 in]
                                n408 = call "Convert to Dynamic Data6"("Array"=w1041) -> ("Dynamic Data Type"=w1065:dynamicdata)  [unwired: 3 in]
                                n409 = Concatenate Strings(w1077, "\\", "File name", "_" ("string"), w1094, "K") -> (w1092:string)
                                n410 = call "Build XY Graph"("Y Input"=w1065, "X Input"=w1066) -> ("XY Graph"=→"R-H":cluster{"X":dbl[], "Y":dbl[]}[])  [unwired: 8 in, 1 out]
                                n411 = String To Path(string=w1092) -> (path=w1076:path)
                                n412 = Format Date/Time String(time format string (%c)="%H:%M:%S%3u") -> (date/time string=w1048:string)  [unwired: 2 in]
                                n413 = Fract/Exp String To Number(string=w1048) -> (number=w1049:dbl)  [unwired: 3 in, 1 out]
                                n414 = Match Pattern(string=w1048, regular expression=":") -> (after substring=w1054:string)  [unwired: 1 in, 3 out]
                                n415 = Fract/Exp String To Number(string=w1054) -> (number=w1056:dbl)  [unwired: 3 in, 1 out]
                                n416 = Match Pattern(string=w1054, regular expression=":") -> (after substring=w1050:string)  [unwired: 1 in, 3 out]
                                n417 = Multiply(x=w1049, y=3600.0) -> (x*y=w1053:dbl)
                                n418 = Fract/Exp String To Number(string=w1050) -> (number=w1047:dbl)  [unwired: 3 in, 1 out]
                                n419 = Multiply(x=w1056, y=60.0) -> (x*y=w1052:dbl)
                                n420 = Add(x=w1053, y=w1052) -> (x+y=w1051:dbl)
                                n421 = Add(x=w1051, y=w1047) -> (x+y=w1046:dbl)
                                n422 = Build Array (concatenate)(w1081, w1091) -> (w1067:dbl[])
                                n423 = Build Array (concatenate)(w1040, w1090) -> (w1069:dbl[])
                                n424 = Build Array (concatenate)(w1089, w1087) -> (w1072:dbl[])
                                n425 = Build Array (concatenate)(w1086, w1046) -> (w1073:dbl[])
                                n426 = call "Convert to Dynamic Data2"("Array"=w1067) -> ("Dynamic Data Type"=w1085:dynamicdata)  [unwired: 3 in]
                                n427 = call "Convert to Dynamic Data3"("Array"=w1069) -> ("Dynamic Data Type"=w1084:dynamicdata)  [unwired: 3 in]
                                n428 = call "Convert to Dynamic Data4"("Array"=w1072) -> ("Dynamic Data Type"=w1083:dynamicdata)  [unwired: 3 in]
                                n429 = call "Convert to Dynamic Data"("Array"=w1073) -> ("Dynamic Data Type"=w1082:dynamicdata)  [unwired: 3 in]
                                n430 = case shown="False" w1035 {
                                tunnel: [w1098 w1108] -> w1088
                                tunnel: w1085 -> [w1101 w1107]
                                tunnel: w1084 -> [_ w1106]
                                tunnel: w1083 -> [w1102 w1105]
                                tunnel: w1082 -> [w1103 w1104]
                                tunnel: w1037 -> [w1100 _]
                                tunnel: w1036 -> [w1099 _]
                                frame False {
                                n431 = Merge Signals(w1101, w1099, w1100, w1102, w1103) -> (w1098:dynamicdata)
                                }
                                frame True {
                                n432 = Merge Signals(w1107, w1106, w1105, w1104) -> (w1108:dynamicdata)
                                }
                                }
                                n433 = case shown="False" "Reset" {
                                tunnel: [w1116 dbl[] []] -> w1074
                                tunnel: w1073 -> [w1116 _]
                                tunnel: w1072 -> [w1115 _]
                                tunnel: [w1115 dbl[] []] -> w1071
                                tunnel: [w1114 dbl[] []] -> w1070
                                tunnel: w1069 -> [w1114 _]
                                tunnel: [w1113 dbl[] []] -> w1068
                                tunnel: w1067 -> [w1113 _]
                                tunnel: w1039 -> [w1112 _]
                                tunnel: [w1111 dbl[] []] -> w1042
                                tunnel: [w1112 dbl[] []] -> w1044
                                tunnel: w1038 -> [w1111 _]
                                frame False {
                                }
                                frame True {
                                }
                                }
                                n434 = call "Write To Measurement File"("Signals"=w1088, "Reset"=TRUE, "Filename"=w1076) -> ("Filename Out"=→"Filename Out":path)  [unwired: 14 in, 2 out]
                                n435 = Build Array (concatenate)(w1042, w1034) -> (w1043:dbl[])
                                n436 = Build Array (concatenate)(w1044, w1033) -> (w1045:dbl[])
                                }
                                frame #5 {
                                n437 = local write "Reset"(FALSE) -> ()
                                }
                                }
                                n438 = call "Time Delay"("Delay Time (s)"="period (s)") -> ()  [unwired: 1 in, 10 out]
                                n439 = case shown="True" w891 {
                                tunnel: [FALSE w1125] -> w879
                                frame False {
                                }
                                frame True {
                                n440 = flat-sequence {
                                tunnel: [TRUE] -> w1125
                                frame #0 {
                                n441 = Multiply(x="Wait field stable [sec]", y=1000.0) -> (x*y=w1126:dbl)
                                n442 = Wait (ms)(milliseconds to wait=w1126) -> ()  [unwired: 1 out]
                                }
                                frame #1 {
                                }
                                }
                                }
                                }
                                n443 = Or(x="Stop", y=w879) -> (x .or. y?=w880:bool)
                                }
                              }
                            }
                          }
                          frame True {
                          }
                        }
                        n444 = Or(x=w757, y=w755) -> (x .or. y?=w756:bool)
                      }
                    }
                  }
                }
              }
            }
            frame True {
            }
          }
          n445 = Or(x=w558, y=w557) -> (x .or. y?=w556:bool)
        }
        n446 = Index Array(array="Set Temp [K]  Rate [K/min]", index (col)=1) -> (element=w549:dbl[])  [unwired: 1 in]
        n447 = Index Array(array="Set Temp [K]  Rate [K/min]", index (col)=0) -> (element=w542:dbl[])  [unwired: 1 in]
        n448 = Array Max & Min(array=w542) -> (max value=w536:dbl, min value=w545:dbl)  [unwired: 2 out]
        n449 = Array Max & Min(array=w549) -> (max value=w547:dbl)  [unwired: 3 out]
        n450 = Less?(x=w545, y=0) -> (x < y?=w546:bool)
        n451 = Greater?(x=w536, y=300) -> (0:w537:bool)
        n452 = Greater?(x=w547, y=100) -> (0:w531:bool)
        n453 = call "Display Message to User"("Enable"=w531) -> ("OK"=w538:bool)  [unwired: 9 in, 1 out]
        n454 = Or(x=w537, y=w546) -> (x .or. y?=w550:bool)
        n455 = call "Display Message to User2"("Enable"=w550) -> ("OK"=w551:bool)  [unwired: 9 in, 1 out]
        n456 = Or(x=w551, y=w538) -> (x .or. y?=w539:bool)
        n457 = Stop(stop? (T)=w539) -> ()
      }
      frame #2 {
        n458 = stacked-sequence {
          tunnel: w1135 -> [w1136 w1139 _ w1157 _ w1162 _]
          tunnel: 0.1 -> [_ _ _ w1147 _ _ _]
          tunnel: 0.0 -> [_ w1137 _ _ _ _ _]
          frame #0 {
            n459 = VISA Clear(VISA resource name=w1136) -> ()  [unwired: 1 in, 2 out]
          }
          frame #1 {
            # "set set field"
            n460 = Number To Fractional String(number=w1137, width (-)=i16 6, precision (6)=i16 3) -> (F-format string=w1142:string)  [unwired: 1 in]
            n461 = Concatenate Strings("S [%][MID] " ("string"), w1142) -> (w1138:string)
            n462 = Concatenate Strings(w1138, "\r") -> (w1141:string)
            n463 = VISA Write(VISA resource name=w1139, write buffer=w1141) -> ()  [unwired: 1 in, 3 out]
          }
          frame #2 {
            n464 = Wait (ms)(milliseconds to wait=500) -> ()  [unwired: 1 out]
          }
          frame #3 {
            # "set rate"
            n465 = Divide(x=w1147, y=60.0) -> (x/y=w1152:dbl)
            n466 = Divide(x=w1152, y=0.09797) -> (x/y=w1150:dbl)
            n467 = Number To Fractional String(number=w1150, width (-)=i16 6, precision (6)=i16 3) -> (F-format string=w1155:string)  [unwired: 1 in]
            n468 = Concatenate Strings("S R " ("string"), w1155) -> (w1154:string)
            n469 = Concatenate Strings(w1154, "\r") -> (w1159:string)
            n470 = VISA Write(VISA resource name=w1157, write buffer=w1159) -> ()  [unwired: 1 in, 3 out]
          }
          frame #4 {
            n471 = Wait (ms)(milliseconds to wait=500) -> ()  [unwired: 1 out]
          }
          frame #5 {
            # "Go to set field"
            n472 = Concatenate Strings("R [%][MID]" ("data"), "\r") -> (w1164:string)
            n473 = VISA Write(VISA resource name=w1162, write buffer=w1164) -> ()  [unwired: 1 in, 3 out]
          }
          frame #6 {
            w1165 = FALSE
            n474 = Wait (ms)(milliseconds to wait=500) -> ()  [unwired: 1 out]
            n475 = local write "Stop"(w1165) -> ()
            n476 = local write "Measure R-H"(w1165) -> ()
          }
        }
      }
    }
  }
